vi "3.24版-复材超声C扫缺陷分析评定软件.vi"() -> ()   [LabVIEW 2018]
doc: "使用该模板构建用户界面事件处理设计模式。将模板应用于对话框及其它用户界面。用户也可创建并执行VI可按照与用户界面事件相同方式处理的用户定义事件。"
uses:
  <vilib>/Utility/NIReport.llb/Report Type.ctl
  <vilib>/addons/_office/_exclsub.llb/font.ctl
  <vilib>/Utility/NIReport.llb/HTML Report Image Alignment.ctl
  <vilib>/Utility/NIReport.llb/Append Report Text (str wrap).vi
  <vilib>/Utility/NIReport.llb/Append Image to Report (path wrap).vi
  <vilib>/addons/_office/word.llb/Word Easy Table (str).vi
  <vilib>/Utility/NIReport.llb/NI_report.lvclass
  <vilib>/vision/NI_Vision_Development_Module.lvlib
  <vilib>/Utility/NIReport.llb/Word/NI_Word.lvclass
  <vilib>/addons/_office/NI_ReportGenerationToolkit.lvlib
  <vilib>/Utility/NIReport.llb/NI_ReportGenerationCore.lvlib
panel:
  out "报告模式":string
  in  "删除标注":bool caption="定量分析"
  out "输入的灰度阈值":dbl caption="值"
  out "反射图原始路径":path
  out "穿透图原始路径":path
  out "ROImask":T1(plugin-control)
  out "模式选择":u16(ring) items=["只读穿透图", "穿透图和反射图结合"]
  out "添加的路径":path
  out "连接的字符串 2":string
  out "临界面积百分比值":dbl
  out "临界Z值":i32
  out "标注后的图片路径":path
  out "弥散类检测结果合并":string[][](table)
  out "分层类检测结果合并":string[][](table)
  out "弥散类检测结果":string[][](table)
  out "分层类检测结果":string[][](table)
  out "部位信息":string[](array[string])=["", "34.500000", "32.500000", "1121", "34", "54.955926", "分层类", "不合格", ""]
  out "连接的字符串":string
  out "框数":dbl
  out "自定义字体":T2={"Desired Font (Application)"=enum."Application Font", "[User-specified Font]"={"Font Name"="", "Size"=12, "Strikeout?"=FALSE, "Italic?"=FALSE, "Underline?"=FALSE, "Outline?"=FALSE, "Shadow?"=FALSE, "Bold?"=FALSE, "Rotation Angle"=0.0}, "Horizontal Alignment"=0, "Vertical Alignment"=0} {"Horizontal Alignment" items=["Left", "Center", "Right"]; "Vertical Alignment" items=["Bottom", "Top", "Baseline"]}
  out "框组":T3(array[cluster])
  out "质量等级":string
  out "灰度阈值":dbl
  in  "stop":bool caption="停止"
  in  "导入图像":bool caption="导入图片"
  in  "图像预处理":bool
  in  "自定义色彩":bool
  in  "开始标注":bool caption="定量分析"
  in  "查看标注":bool caption="辅助定性分析"
  in  "生成评定结果":bool caption="生成原始记录"
  in  "控件":enum32{"穿透图", "反射图"}(tab)
  out "穿透图":T1(plugin-control)
  out "反射图":T1(plugin-control)
  out "产品规格":cluster{"产品长度（周长）（mm）":dbl, "产品宽度（母线长）（mm）":dbl}
  out "图像分辨率":T4
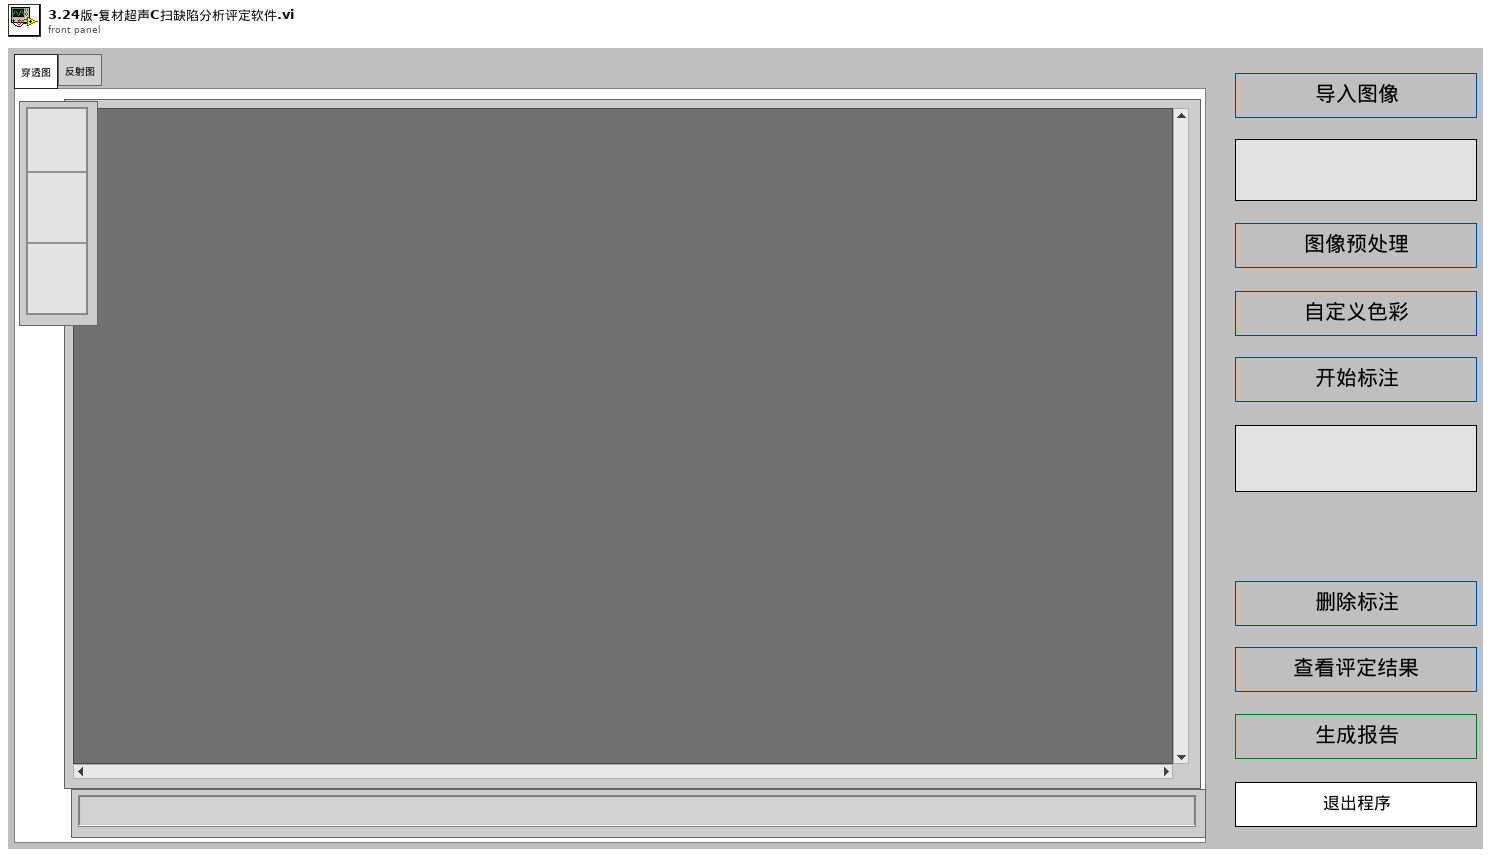
[diagram p1: front panel]
types:
  T1 = typedef "IMAQ Image.ctl" = refnum<image>
  T2 = cluster{"Desired Font (Application)":enum16{"User-specified Font", "Application Font", "System Font", "Dialog Font"}, "[User-specified Font]":cluster{"Font Name":string, "Size":i16, "Strikeout?":bool, "Italic?":bool, "Underline?":bool, "Outline?":bool, "Shadow?":bool, "Bold?":bool, "Rotation Angle":dbl}, "Horizontal Alignment":i16, "Vertical Alignment":i16}
  T3 = cluster{"Global Rectangle":i32[], "Contours":cluster{"Contour Type":u32, "ROI Type":u32, "Points":i32[]}[]}[]
  T4 = cluster{"图像X向分辨率（mm/像素）":dbl, "图像Y向分辨率（mm/像素）":dbl}
  T5 = cluster{"Global Rectangle":i32[], "Contours":cluster{"Contour Type":u32, "ROI Type":u32, "Points":i32[]}[]}
  T6 = cluster{"Zoom Tool":bool, "Selection Tool":bool, "Pan Tool":bool, "Point Tool":bool, "Line Tool":bool, "Rectangle Tool":bool, "Rotated Rectangle Tool":bool, "Polyline Tool":bool, "Polygon Tool":bool, "Freehand Tool":bool, "Closed Freehand Tool":bool, "Ellipse Tool":bool, "Annulus Tool":bool}
  T7 = enum8{"Enabled", "Disabled", "Disabled and Grayed Out"}
  T8 = enum32{"Invalid", "Standard", "Closed", "Hidden", "Minimized", "Maximized"}
  T9 = enum32{"Linear", "Log", "Exp", "Square", "Square root", "Power X", "Power 1/X"}
  T10 = enum32{"Gray", "Binary", "Gradient", "Rainbow", "Temperature"}
  T11 = enum16{"maximized", "minimized", "normal", "no change"}
  T12 = typedef "NI_ReportGenerationCore.lvlib/Report Type.ctl" = enum16{"HTML", "Word", "Excel"}
  T13 = typedef "NI_ReportGenerationCore.lvlib/HTML Report Image Alignment.ctl" = enum16{"(default)", "LEFT", "RIGHT", "TOP", "TEXTTOP", "MIDDLE", "ABSMIDDLE", "BASELINE", "BOTTOM", "ABSBOTTOM"}
  T14 = cluster{"position (Excel)":cluster{"row":i32, "column":i32}, "name (Excel)":string, "bookmark (Word)":string}
  T15 = cluster{"position (excel)":cluster{"row":i32, "column":i32}, "name (excel)":string, "bookmark (word)":string}
  T16 = typedef "NI_ReportGenerationToolkit.lvlib/font.ctl" = cluster{"font name":string, "font size":dbl, "bold":u16, "italic":u16, "underline":u16, "strike through":u16, "font color":u32}
  T17 = typedef "Image Type" = u32
  T18 = cluster{"Red (or Hue) value":u8, "Green (or Sat) value":u8, "Blue (or Light or Val) value":u8}[]
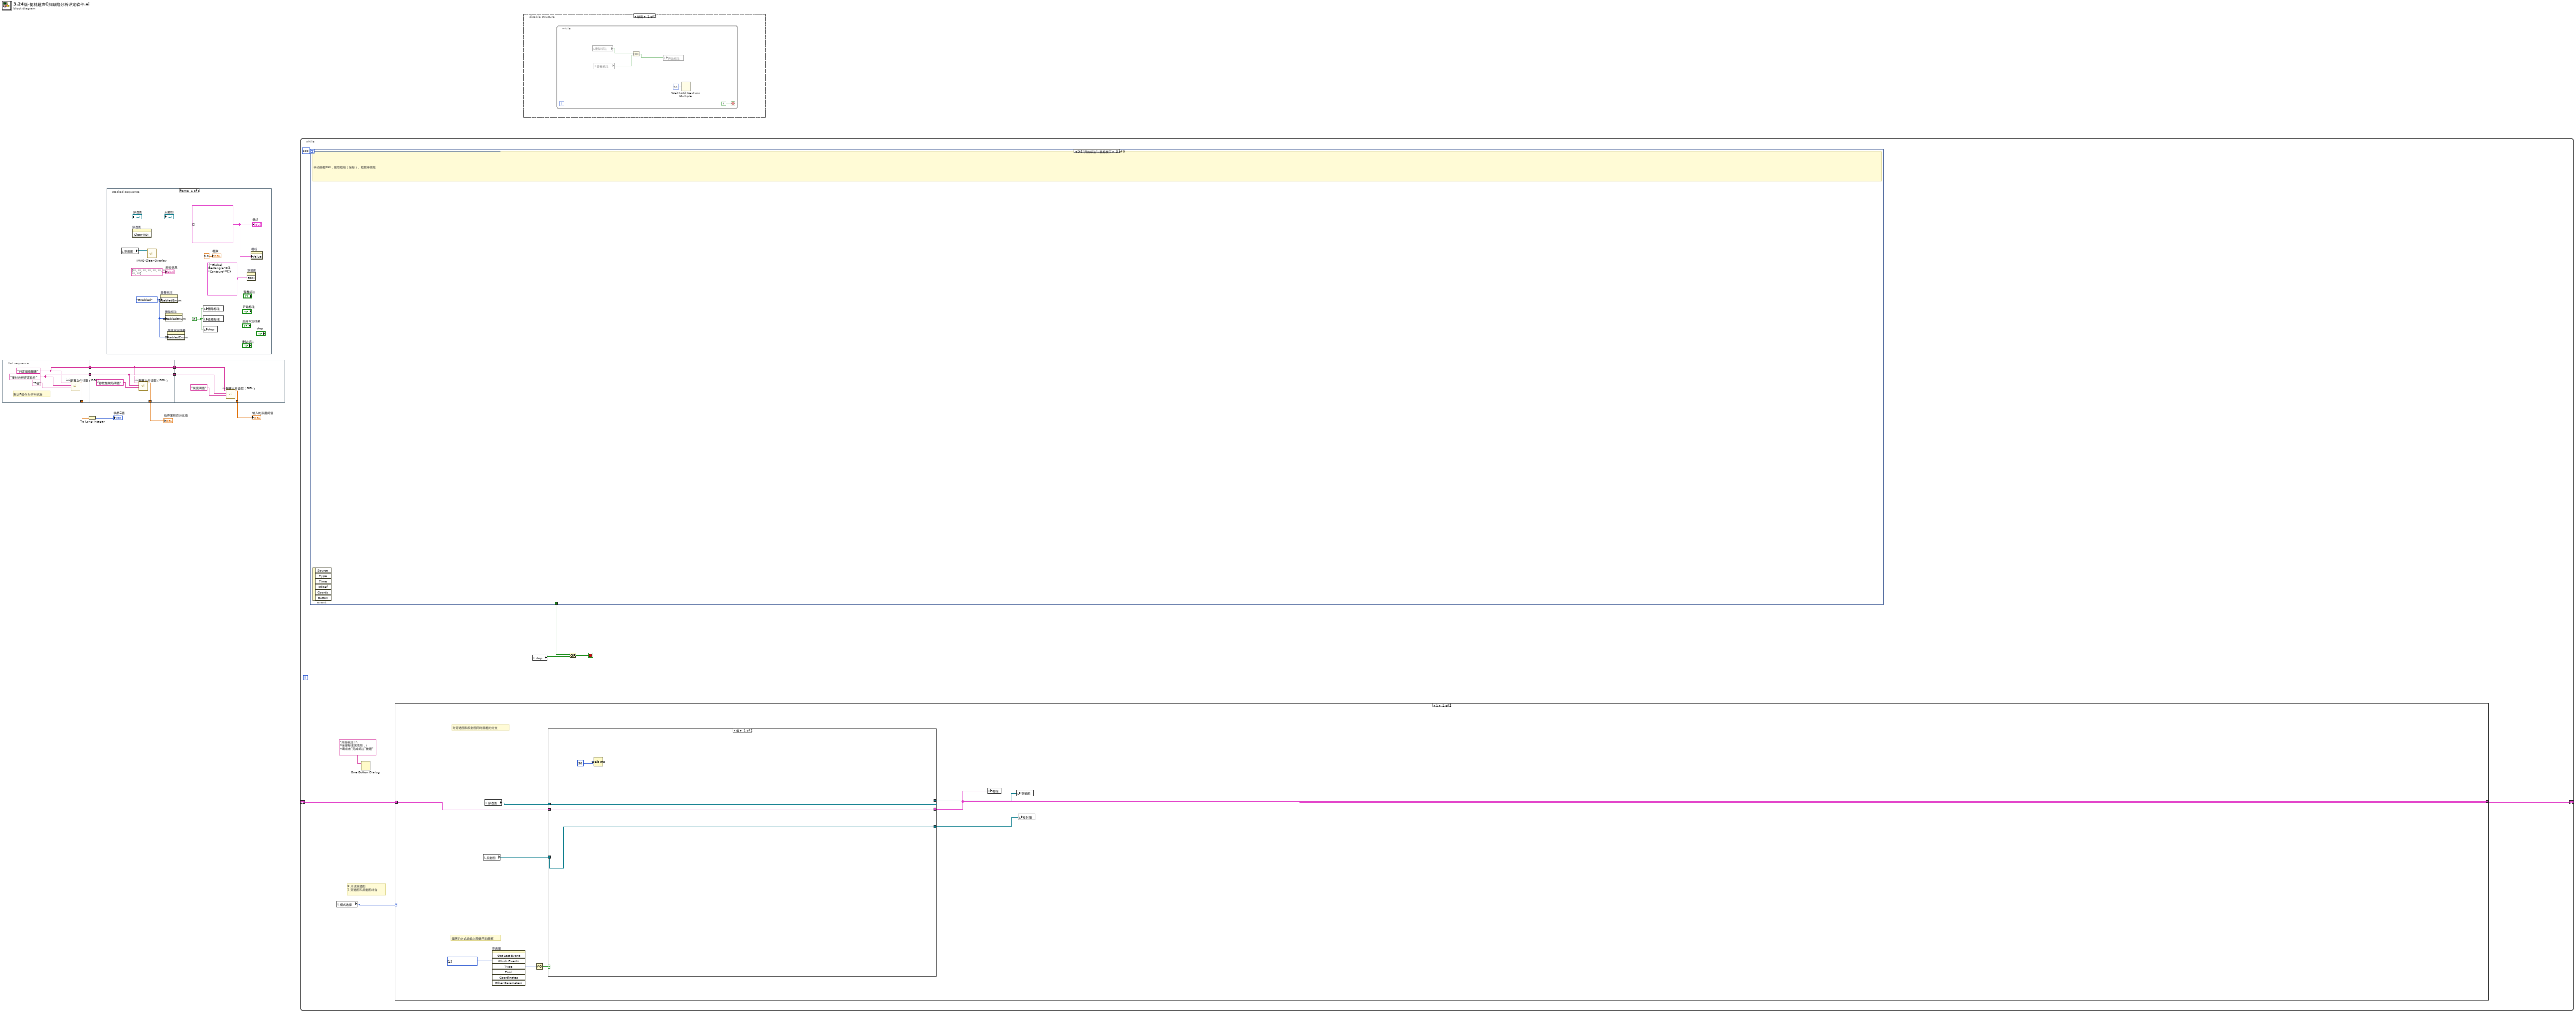
[diagram p0: block diagram]
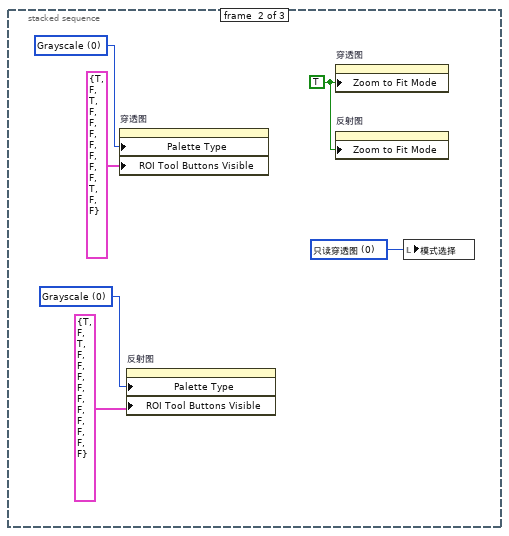
[diagram p2: hidden frame]
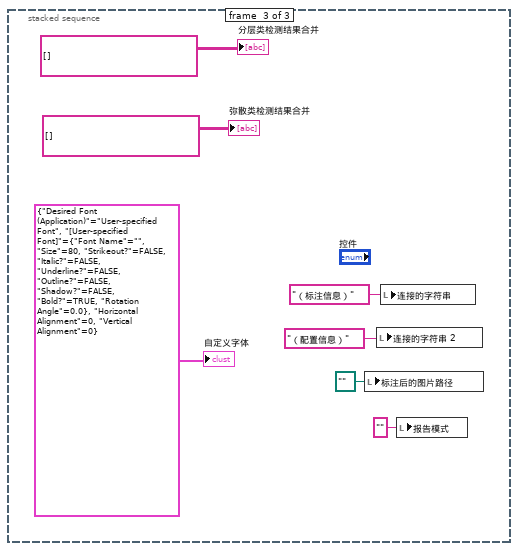
[diagram p3: hidden frame]
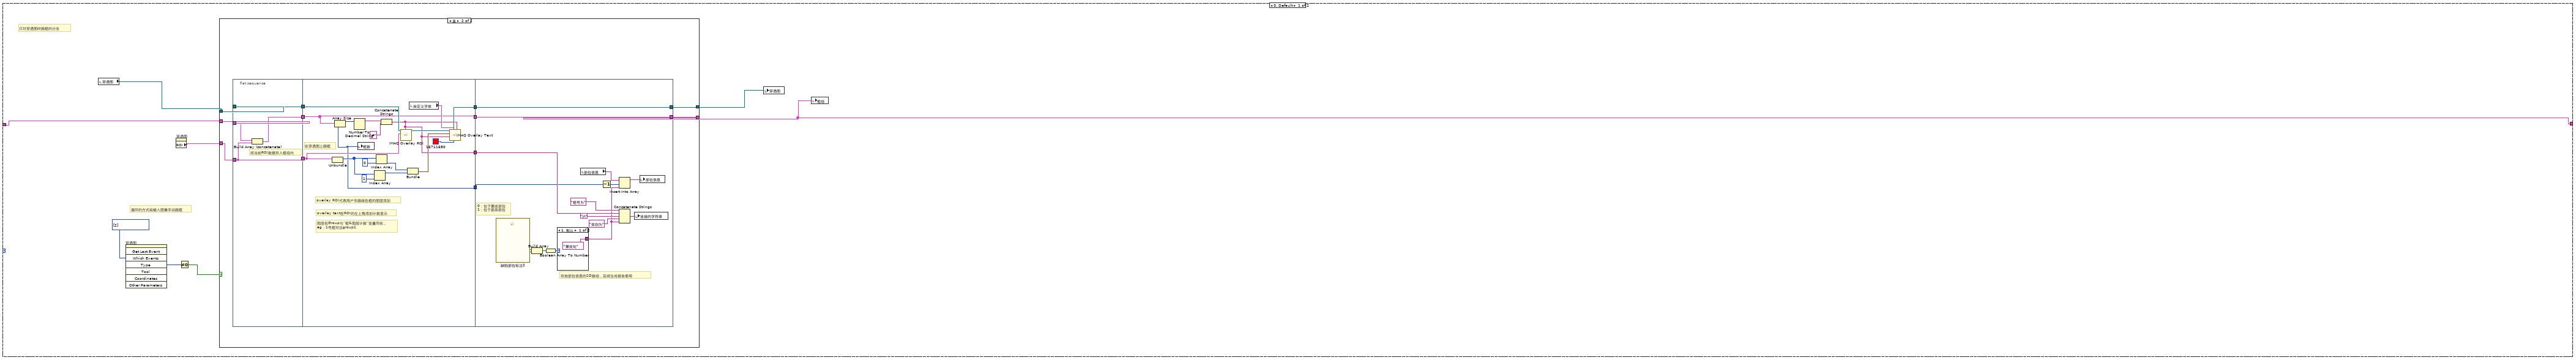
[diagram p5: hidden frame]
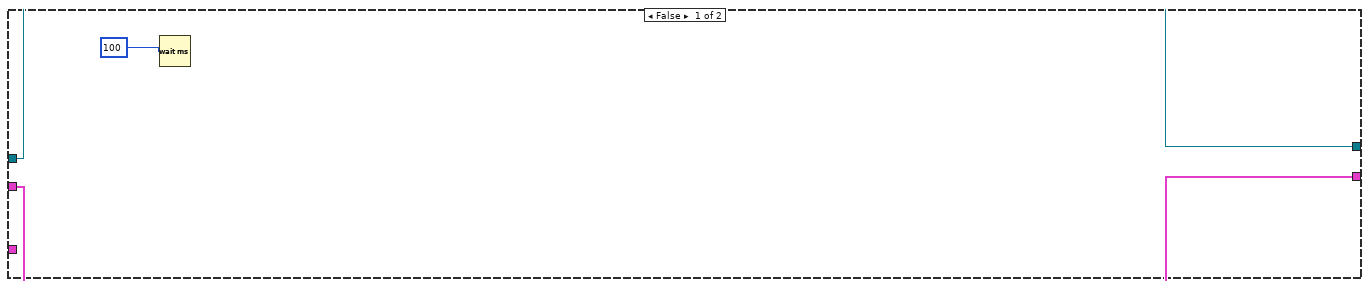
[diagram p6: hidden frame]
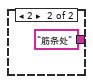
[diagram p7: hidden frame]
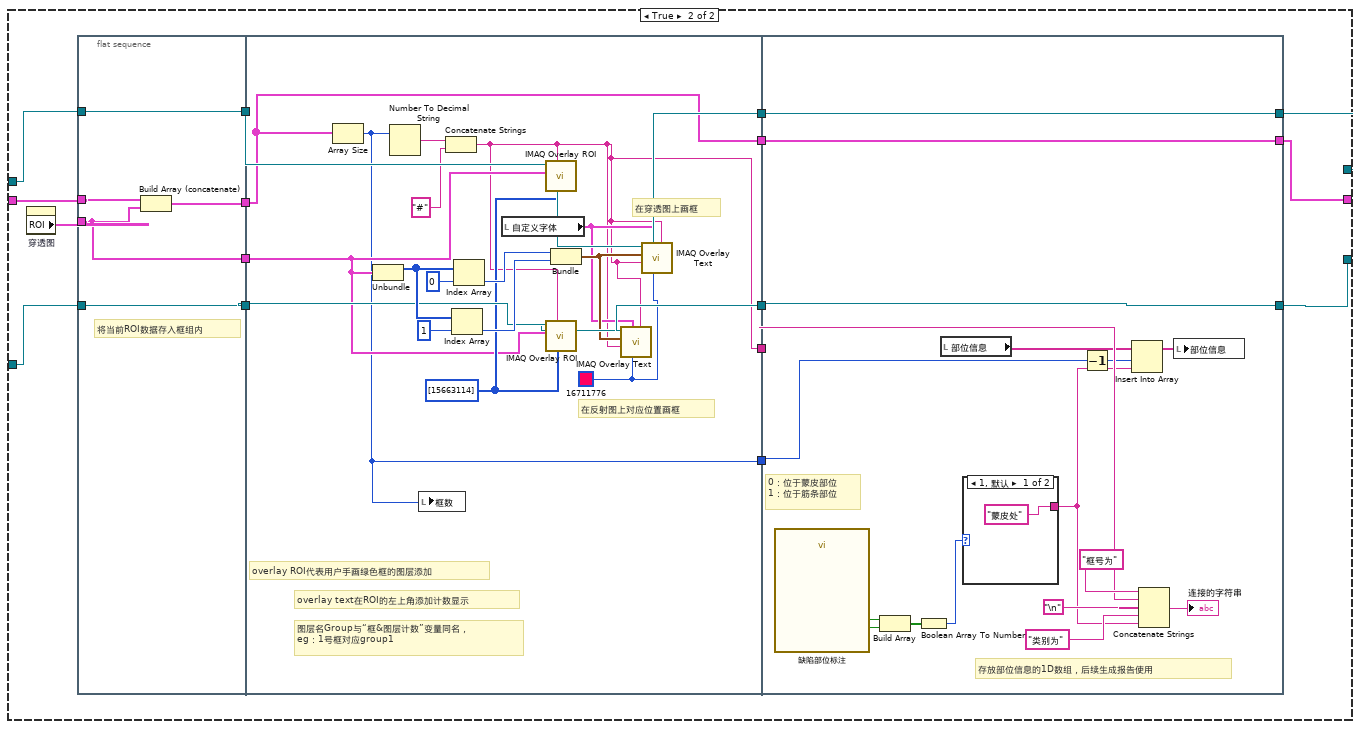
[diagram p8: hidden frame]
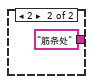
[diagram p9: hidden frame]
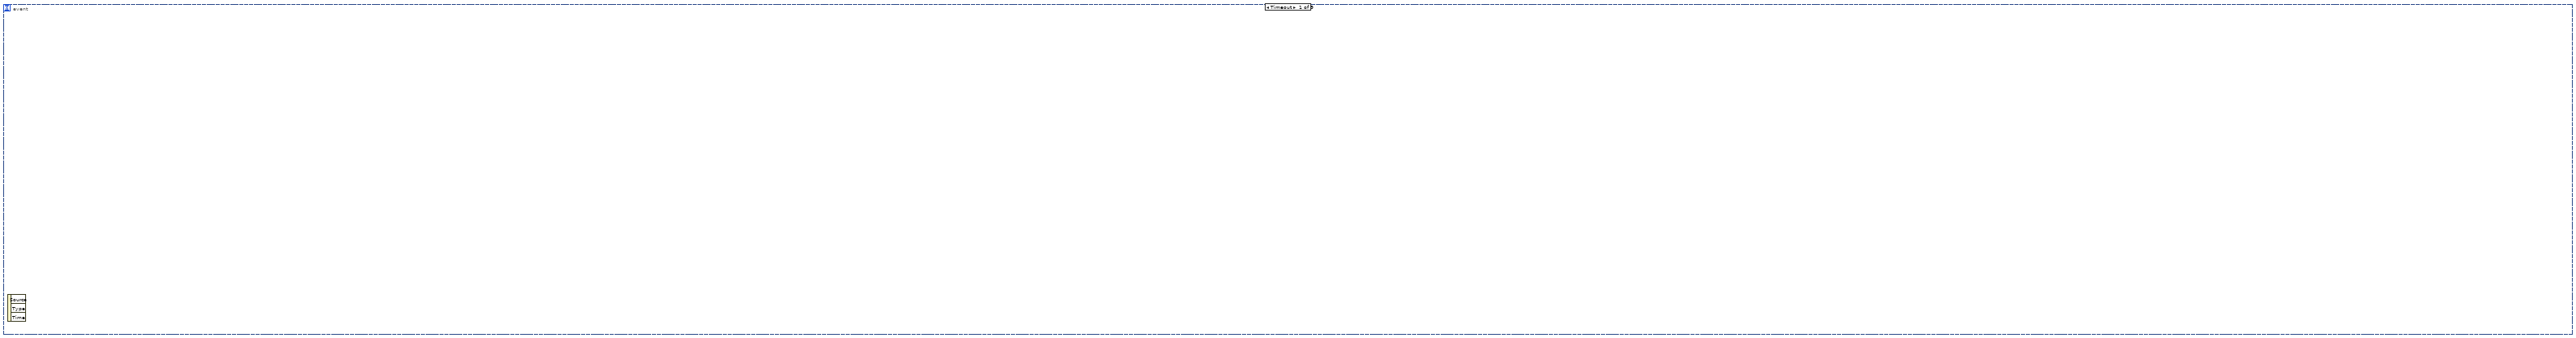
[diagram p10: hidden frame]
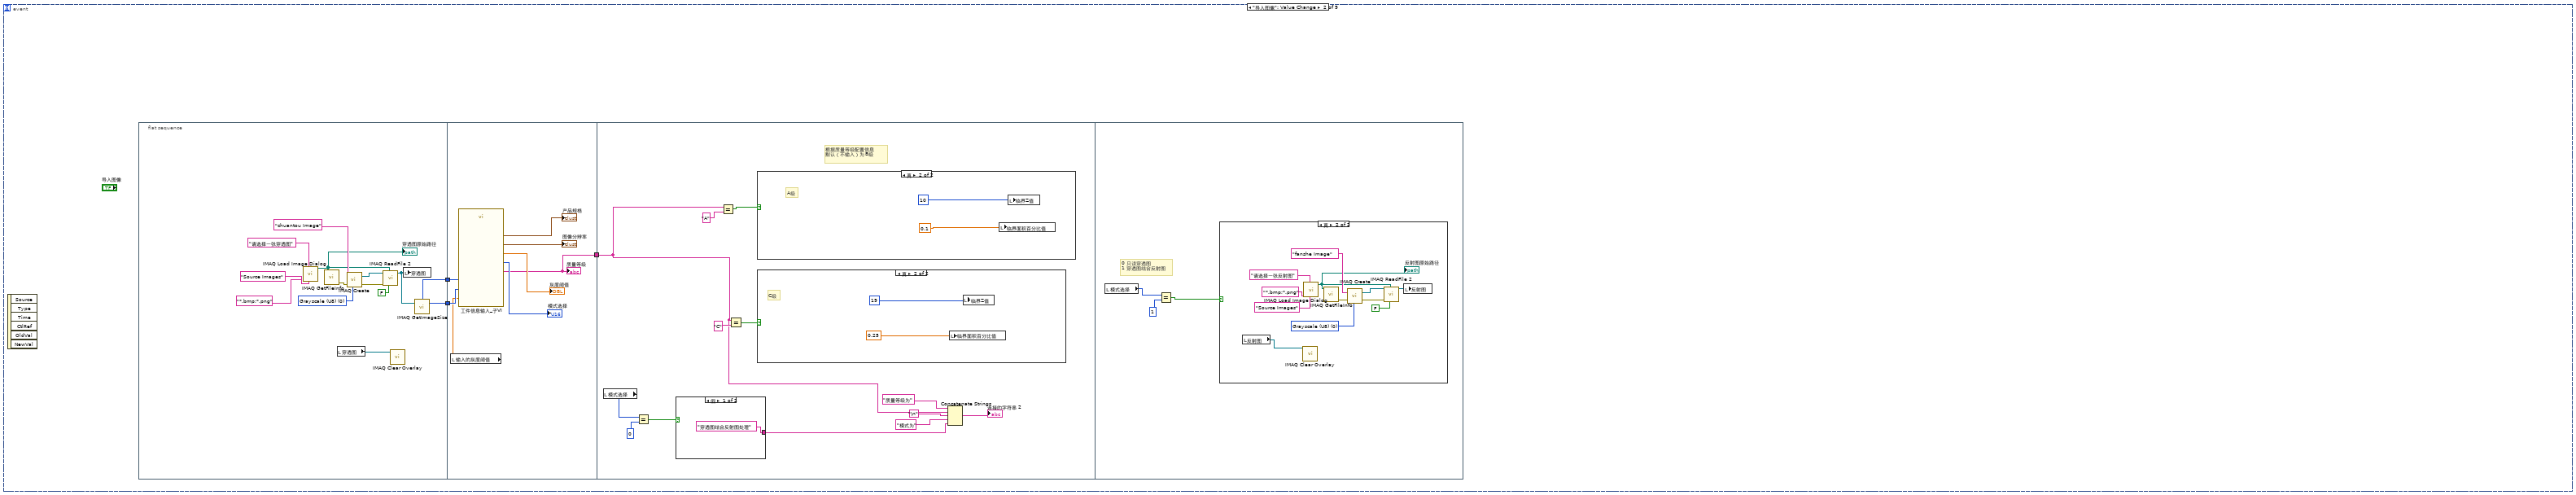
[diagram p11: hidden frame]
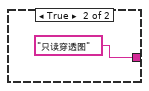
[diagram p12: hidden frame]
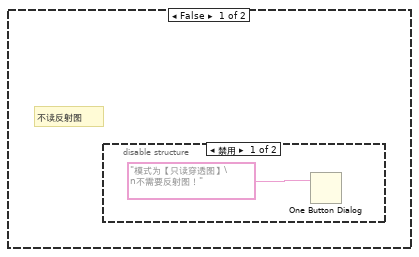
[diagram p15: hidden frame]
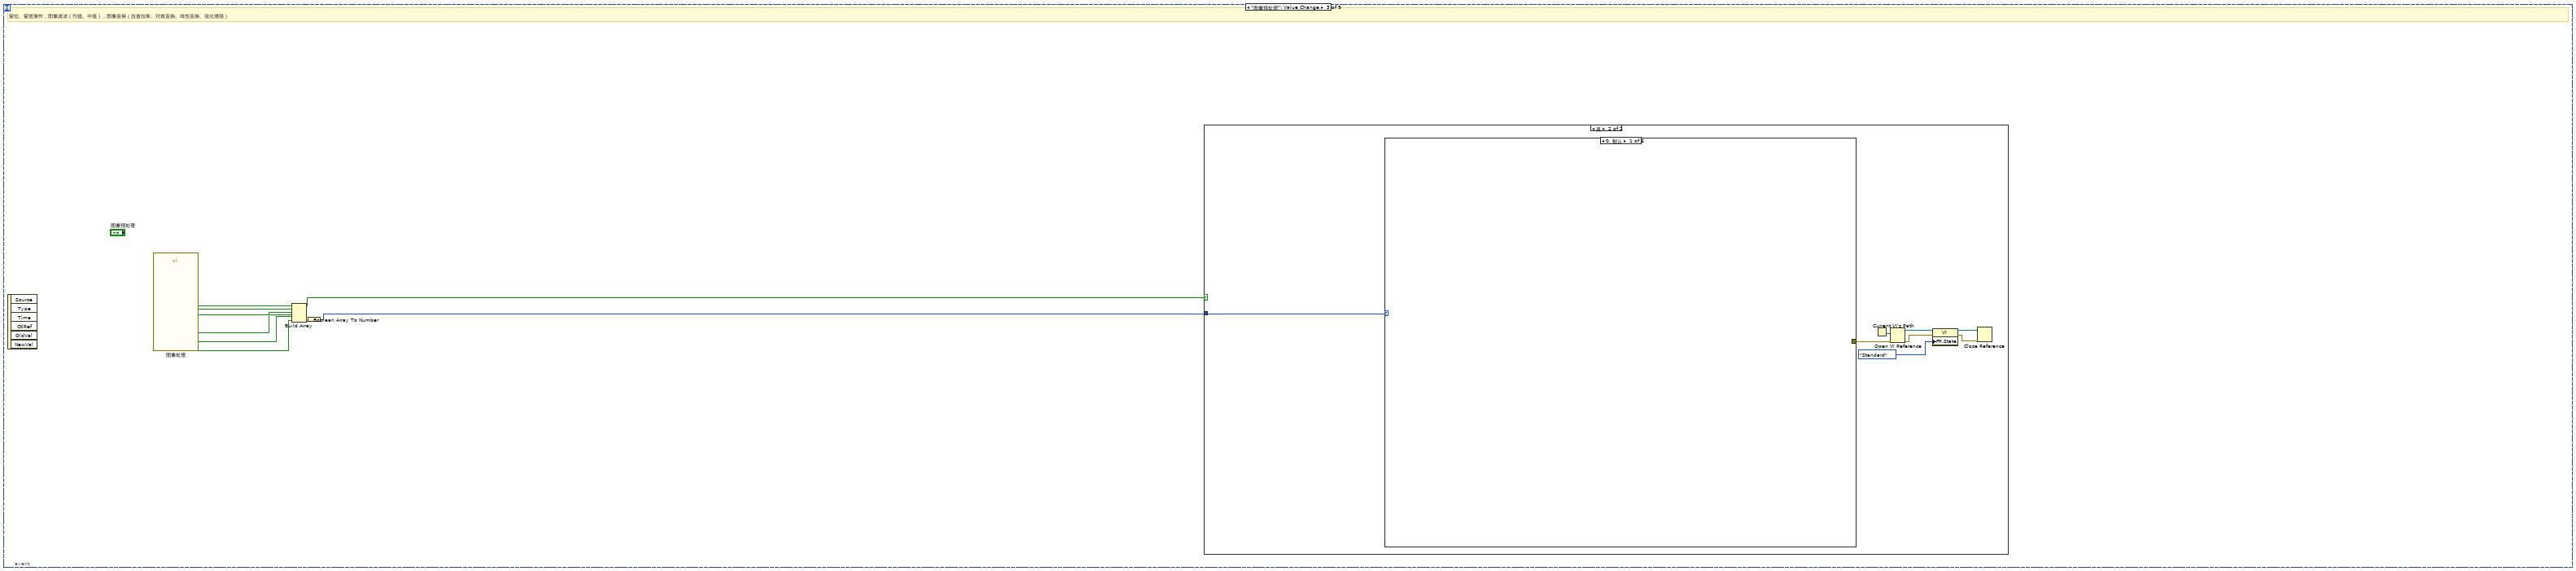
[diagram p17: hidden frame]
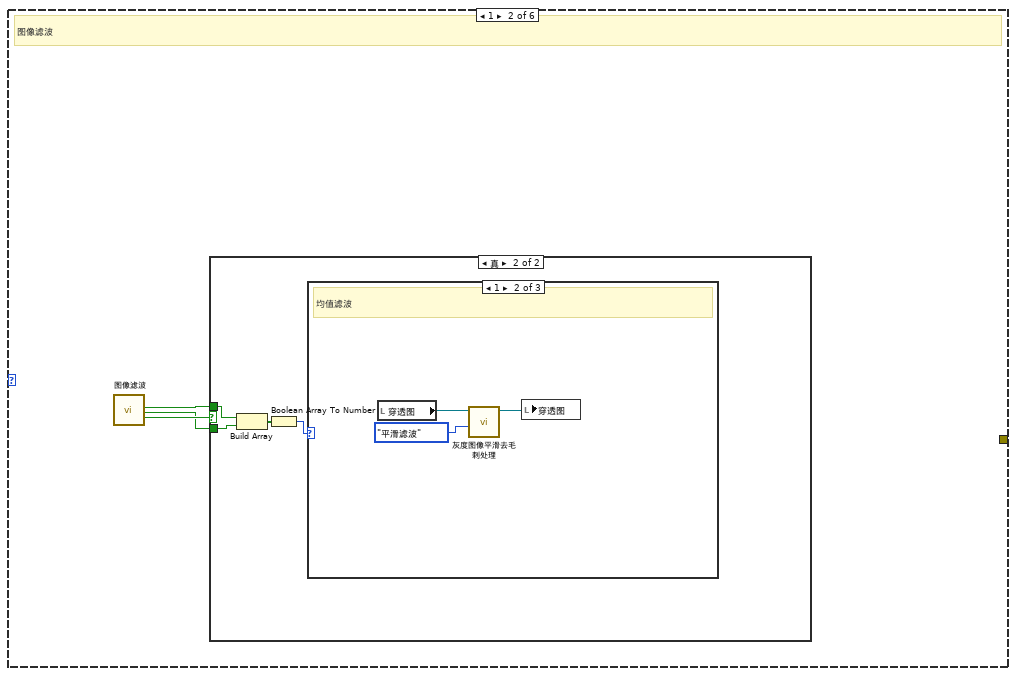
[diagram p19: hidden frame]
diagram:
  n1 = flat-sequence {
    tunnel: [w11] -> w8
    tunnel: [w10] -> w7
    tunnel: [w9] -> w2
    tunnel: w8 -> [w14]
    tunnel: w7 -> [w15]
    tunnel: [w15] -> w6
    tunnel: [w14] -> w5
    tunnel: [w13] -> w3
    tunnel: w6 -> [w19]
    tunnel: w5 -> [w18]
    tunnel: [w17] -> w4
    frame #0 {
      w10 = "复材分析评定软件" ("section")
      w11 = "判定阈值配置" ("文件名称")
      # "默认B级作为评判标准"
      n2 = call "ini配置文件读取（DBL）.vi"("key"="Z值", "section"=w10, "文件名称"=w11) -> ("value"=w9:dbl)  [unwired: 8 in]
    }
    frame #1 {
      n3 = call "ini配置文件读取（DBL）.vi"("key"="弥散性缺陷阈值", "section"=w15, "文件名称"=w14) -> ("value"=w13:dbl)  [unwired: 8 in]
    }
    frame #2 {
      n4 = call "ini配置文件读取（DBL）.vi"("key"="灰度阈值", "section"=w19, "文件名称"=w18) -> ("value"=w17:dbl)  [unwired: 8 in]
    }
  }
  n5 = To Long Integer(number=w2) -> (32bit integer=→"临界Z值":i32)
  n6 = stacked-sequence {
    frame #0 {
      w25 = T3 [] ("框组")
      w22 = T7."Enabled" ("禁用")
      w21 = FALSE ("查看标注")
      n7 = local read "穿透图"() -> (w23:T1)
      n8 = invoke on="穿透图" class="ImageControl" method="Clear ROI"() -> ()  [unwired: 3 in, 3 out]
      n9 = call "IMAQ Clear Overlay"("Image"=w23) -> ()  [unwired: 9 in, 2 out]
      n10 = property on="查看标注" class="Bool (严格)"("DisabledEnum"=w22) -> ()  [unwired: 2 in, 2 out]
      n11 = property on="删除标注" class="Bool (严格)"("DisabledEnum"=w22) -> ()  [unwired: 2 in, 2 out]
      n12 = property on="生成评定结果" class="Bool"("DisabledEnum"=w22) -> ()  [unwired: 2 in, 2 out]
      n13 = local write "删除标注"(w21) -> ()
      n14 = local write "查看标注"(w21) -> ()
      n15 = local write "stop"(w21) -> ()
      n16 = property on="穿透图" class="ImageControl"("ROI"=T5 {"Global Rectangle"=[], "Contours"=[]}) -> ()  [unwired: 2 in, 2 out]
      n17 = property on="框组" class="Arr (严格)"("Value"=w25) -> ()  [unwired: 2 in, 2 out]
      "部位信息" <- string[] ["", "", "", "", "", "", "", "", ""] ("部位信息")
      "框组" <- w25
      "框数" <- 0.0 ("框数")
    }
    frame #1 {
      w28 = u16 0 items=["只读穿透图", "穿透图和反射图结合"] ("模式选择")
      w30 = u32 0 items=["Grayscale", "Binary", "Gradient", "Rainbow", "Temperature", "User Defined", "Binary 16 Bit", "Gradient 16 Bit", "Rainbow 16 Bit", "Temperature 16 Bit", "User Defined 16 Bit"] ("Palette:Palette Type")
      w31 = TRUE ("Zoom to Fit Mode")
      w33 = u32 0 items=["Grayscale", "Binary", "Gradient", "Rainbow", "Temperature", "User Defined", "Binary 16 Bit", "Gradient 16 Bit", "Rainbow 16 Bit", "Temperature 16 Bit", "User Defined 16 Bit"] ("Palette:Palette Type")
      n18 = property on="穿透图" class="ImageControl"("Palette Type"=w33, "ROI Tool Buttons Visible"=T6 {"Zoom Tool"=TRUE, "Selection Tool"=FALSE, "Pan Tool"=TRUE, "Point Tool"=FALSE, "Line Tool"=FALSE, "Rectangle Tool"=FALSE, "Rotated Rectangle Tool"=FALSE, "Polyline Tool"=FALSE, "Polygon Tool"=FALSE, "Freehand Tool"=FALSE, "Closed Freehand Tool"=TRUE, "Ellipse Tool"=FALSE, "Annulus Tool"=FALSE} ("ROI Tool Buttons Visible:All Elements")) -> ()  [unwired: 2 in, 2 out]
      n19 = property on="反射图" class="ImageControl"("Palette Type"=w30, "ROI Tool Buttons Visible"=T6 {"Zoom Tool"=TRUE, "Selection Tool"=FALSE, "Pan Tool"=TRUE, "Point Tool"=FALSE, "Line Tool"=FALSE, "Rectangle Tool"=FALSE, "Rotated Rectangle Tool"=FALSE, "Polyline Tool"=FALSE, "Polygon Tool"=FALSE, "Freehand Tool"=FALSE, "Closed Freehand Tool"=FALSE, "Ellipse Tool"=FALSE, "Annulus Tool"=FALSE} ("ROI Tool Buttons Visible:All Elements")) -> ()  [unwired: 2 in, 2 out]
      n20 = property on="穿透图" class="ImageControl"("Zoom to Fit Mode"=w31) -> ()  [unwired: 2 in, 2 out]
      n21 = property on="反射图" class="ImageControl"("Zoom to Fit Mode"=w31) -> ()  [unwired: 2 in, 2 out]
      n22 = local write "模式选择"(w28) -> ()
    }
    frame #2 {
      n23 = local write "标注后的图片路径"(path "" ("标注后的图片路径")) -> ()
      n24 = local write "连接的字符串 2"("（配置信息）" ("连接的字符串 2")) -> ()
      n25 = local write "连接的字符串"("（标注信息）" ("连接的字符串")) -> ()
      n26 = local write "报告模式"("" ("报告模式")) -> ()
      "自定义字体" <- T2 {"Desired Font (Application)"=enum."User-specified Font", "[User-specified Font]"={"Font Name"="", "Size"=80, "Strikeout?"=FALSE, "Italic?"=FALSE, "Underline?"=FALSE, "Outline?"=FALSE, "Shadow?"=FALSE, "Bold?"=TRUE, "Rotation Angle"=0.0}, "Horizontal Alignment"=0, "Vertical Alignment"=0} ("Font, Size & Style")
      "分层类检测结果合并" <- string[][] [] ("弥散类检测结果合并")
      "弥散类检测结果合并" <- string[][] [] ("弥散类检测结果合并")
    }
  }
  n27 = while {
    shift-right: [w44] -> _
    shift-left: _ -> [w45]
    stop <- w41 stop-if-true
    # "0 只读穿透图\n1 穿透图和反射图结合"
    n28 = event shown="[4] \"开始标注\": 鼠标按下" {
      selector: _ -> [_ _ _ _ _ _ _ _ _]
      dyn-events: _ -> [_ _ _ _ _ _ _ _ _]
      timeout: 100 -> [_ _ _ _ _ _ _ _ _]
      tunnel: [_ _ _ _ _ _ _ _ w763] -> w42
      event Timeout {
        n29 = event-data() -> ()  [unwired: 1 in, 3 out]
      }
      event "导入图像": Value Change {
        n30 = event-data() -> ()  [unwired: 1 in, 6 out]
        n31 = flat-sequence {
          tunnel: [w191] -> w187
          tunnel: [w190] -> w186
          tunnel: [w206] -> w188
          tunnel: w187 -> [w205]
          tunnel: w186 -> [w204]
          tunnel: w188 -> [w215]
          frame #0 {
            w194 = T17 0 items=["Grayscale (U8)", "Grayscale (I16)", "Grayscale (SGL)", "Complex (CSG)", "RGB (U32)", "HSL (U32)", "RGB (U64)", "Grayscale (U16)"] ("Image Type")
            n32 = call "IMAQ Load Image Dialog"("Pattern Label"="Source Images", "Prompt"="请选择一张穿透图" ("prompt"), "Pattern"="*.bmp;*.png") -> ("Path"=w193:path)  [unwired: 6 in, 2 out]
            "穿透图原始路径" <- w193
            n33 = call "IMAQ GetFileInfo"("File Path"=w193) -> ("error out"=w197:errorcluster)  [unwired: 4 in, 6 out]
            n34 = local read "穿透图"() -> (w189:T1)
            n35 = call "IMAQ Create"("Image Name"="chuantou Image", "Image Type"=w194, "error in (no error)"=w197) -> ("New Image"=w198:T1, "error out"=w199:errorcluster)  [unwired: 2 in]
            n36 = call "IMAQ ReadFile 2"("Use File Path Image Type"=FALSE, "File Path"=w193, "error in (no error)"=w199, "Image"=w198) -> ("Image Out"=w192:T1)  [unwired: 3 in, 4 out]
            n37 = call "IMAQ Clear Overlay"("Image"=w189) -> ()  [unwired: 9 in, 2 out]
            n38 = local write "穿透图"(w192) -> ()
            n39 = call "IMAQ GetImageSize"("Image"=w192) -> ("Y Resolution"=w190:i32, "X Resolution"=w191:i32)  [unwired: 3 in, 1 out]
          }
          frame #1 {
            n40 = local read "输入的灰度阈值"() -> (w203:dbl)
            n41 = call "工件信息输入_子VI.vi"("Y Resolution"=w204, "X Resolution"=w205, "输入的灰度阈值"=w203) -> ("质量等级"=w206:string, "模式选择"=→"模式选择":u16, "灰度阈值"=→"灰度阈值":dbl, "产品规格"=→"产品规格":cluster{"产品长度（周长）（mm）":dbl, "产品宽度（母线长）（mm）":dbl}, "图像分辨率"=→"图像分辨率":T4)  [unwired: 3 in]
            "质量等级" <- w206
          }
          frame #2 {
            # "根据质量等级配置信息\n默认（不输入）为B级"
            n42 = local read "模式选择"() -> (w213:u16)
            n43 = Equal?(x=w213, y=u16 0) -> (x = y?=w212:bool)
            n44 = case shown="假" w212 {
              tunnel: ["穿透图结合反射图处理" ("字符串") "只读穿透图" ("字符串")] -> w211
              frame False {
              }
              frame True {
              }
            }
            n45 = Equal?(x=w215, y="A") -> (x = y?=w218:bool)
            n46 = Equal?(x=w215, y="C") -> (x = y?=w219:bool)
            n47 = case shown="真" w218 {
              frame False {
              }
              frame True {
                # "A级"
                n48 = local write "临界面积百分比值"(0.1 ("临界面积百分比值")) -> ()
                n49 = local write "临界Z值"(10 ("临界Z值")) -> ()
              }
            }
            n50 = case shown="真" w219 {
              frame False {
              }
              frame True {
                # "C级"
                n51 = local write "临界面积百分比值"(0.25 ("临界面积百分比值")) -> ()
                n52 = local write "临界Z值"(19 ("临界Z值")) -> ()
              }
            }
            n53 = Concatenate Strings("质量等级为" ("字符串"), w215, "\n", "模式为" ("字符串"), w211) -> (→"连接的字符串 2":string)
          }
          frame #3 {
            # "0 只读穿透图\n1 穿透图结合反射图"
            n54 = local read "模式选择"() -> (w231:u16)
            n55 = Equal?(x=w231, y=u16 1) -> (x = y?=w230:bool)
            n56 = case shown="真" w230 {
              frame False {
                # "不读反射图"
                n57 = disable-structure shown="禁用" {
                  frame Disabled {
                    n58 = One Button Dialog(message="模式为【只读穿透图】\n不需要反射图！" ("消息")) -> ()  [unwired: 1 in, 1 out]
                  }
                  frame Enabled {
                  }
                }
              }
              frame True {
                w237 = T17 0 items=["Grayscale (U8)", "Grayscale (I16)", "Grayscale (SGL)", "Complex (CSG)", "RGB (U32)", "HSL (U32)", "RGB (U64)", "Grayscale (U16)"] ("Image Type")
                n59 = local read "反射图"() -> (w234:T1)
                n60 = call "IMAQ Clear Overlay"("Image"=w234) -> ()  [unwired: 9 in, 2 out]
                n61 = call "IMAQ Load Image Dialog"("Pattern Label"="Source Images", "Prompt"="请选择一张反射图" ("prompt"), "Pattern"="*.bmp;*.png") -> ("Path"=w236:path)  [unwired: 6 in, 2 out]
                "反射图原始路径" <- w236
                n62 = call "IMAQ GetFileInfo"("File Path"=w236) -> ("error out"=w240:errorcluster)  [unwired: 4 in, 6 out]
                n63 = call "IMAQ Create"("Image Name"="fanshe Image", "Image Type"=w237, "error in (no error)"=w240) -> ("New Image"=w241:T1, "error out"=w242:errorcluster)  [unwired: 2 in]
                n64 = call "IMAQ ReadFile 2"("Use File Path Image Type"=FALSE, "File Path"=w236, "error in (no error)"=w242, "Image"=w241) -> ("Image Out"=w235:T1)  [unwired: 3 in, 4 out]
                n65 = local write "反射图"(w235) -> ()
              }
            }
          }
        }
      }
      event "图像预处理": Value Change {
        # "窗位、窗宽操作，图像滤波（均值、中值），图像变换（拉普拉斯、对数变换、线性变换、锐化增强）"
        n66 = event-data() -> ()  [unwired: 1 in, 6 out]
        n67 = call "图像处理"() -> ("撤销图像处理"=w246:bool, "线性灰度值测量"=w247:bool, "窗位窗宽"=w252:bool, "图像增强"=w248:bool, "图像滤波"=w253:bool, "确定"=w249:bool)  [unwired: 13 in, 1 out]
        n68 = Build Array(w253, w248, w252, w247, w246) -> (w251:bool[])
        n69 = Boolean Array To Number(Boolean array=w251) -> (number=w250:u32)
        n70 = case shown="真" w249 {
          tunnel: w250 -> [_ w261]
          frame False {
          }
          frame True {
            n71 = case shown="0, 默认" w261 {
              tunnel: [_ _ errorcluster {"status"=FALSE, "code"=0, "source"=""} ("错误输入（无错误）") _ _ _] -> w254
              frame 0, Default {
              }
              frame 1 {
                # "图像滤波"
                n72 = call "图像滤波"() -> ("均值滤波"=w263:bool, "中值滤波"=w262:bool, "确定"=w264:bool)  [unwired: 16 in, 1 out]
                n73 = case shown="真" w264 {
                  tunnel: w263 -> [_ w267]
                  tunnel: w262 -> [_ w266]
                  frame False {
                  }
                  frame True {
                    n74 = Build Array(w267, w266) -> (w268:bool[])
                    n75 = Boolean Array To Number(Boolean array=w268) -> (number=w265:u32)
                    n76 = case shown="1" w265 {
                      frame 0, Default {
                      }
                      frame 1 {
                        # "均值滤波"
                        n77 = local read "穿透图"() -> (w271:T1)
                        n78 = call "灰度图像平滑去毛刺处理.vi"("滤波方法选择"=enum16{"中值滤波", "平滑滤波"}."平滑滤波", "Image"=w271) -> ("Image Out"=w270:T1)  [unwired: 9 in]
                        n79 = local write "穿透图"(w270) -> ()
                      }
                      frame 2 {
                        # "中值滤波"
                        n80 = local read "穿透图"() -> (w274:T1)
                        n81 = call "灰度图像平滑去毛刺处理.vi"("滤波方法选择"=enum16{"中值滤波", "平滑滤波"}."中值滤波", "Image"=w274) -> ("Image Out"=w273:T1)  [unwired: 9 in]
                        n82 = local write "穿透图"(w273) -> ()
                      }
                    }
                  }
                }
              }
              frame 2 {
                # "图像增强"
                n83 = call "图像增强"() -> ("幂变换"=w276:bool, "阈值变换"=w277:bool, "高斯变换"=w278:bool, "指数变换"=w279:bool, "对数变换"=w280:bool, "确定"=w281:bool)  [unwired: 13 in, 1 out]
                n84 = case shown="真" w281 {
                  tunnel: w280 -> [_ w286]
                  tunnel: w279 -> [_ w285]
                  tunnel: w278 -> [_ w284]
                  tunnel: w277 -> [_ w283]
                  tunnel: w276 -> [_ w282]
                  frame False {
                  }
                  frame True {
                    n85 = Build Array(w286, w285, w284, w283, w282) -> (w288:bool[])
                    n86 = Boolean Array To Number(Boolean array=w288) -> (number=w287:u32)
                    n87 = case shown="2" w287 {
                      frame 0, Default {
                      }
                      frame 1 {
                        # "对数变换"
                        n88 = call "对数变换"() -> ("变换系数K"=w289:dbl, "确定"=w290:bool)  [unwired: 17 in, 1 out]
                        n89 = case shown="真" w290 {
                          tunnel: w289 -> [_ w291]
                          frame False {
                          }
                          frame True {
                            n90 = local read "穿透图"() -> (w295:T1)
                            n91 = call "IMAQ MathLookup"("Range"=cluster{"Minimum":sgl, "Maximum":sgl} {"Minimum"=0.0, "Maximum"=255.0}, "Operator"=T9."Log", "X Value"=w291, "Image Dst"=w295, "Image Src"=w295) -> ("Image Dst Out"=w293:T1)  [unwired: 5 in, 1 out]
                            n92 = local write "穿透图"(w293) -> ()
                          }
                        }
                      }
                      frame 2 {
                        # "指数变换"
                        n93 = call "指数变换"() -> ("变换系数K"=w296:dbl, "确定"=w297:bool)  [unwired: 17 in, 1 out]
                        n94 = case shown="真" w297 {
                          tunnel: w296 -> [_ w298]
                          frame False {
                          }
                          frame True {
                            n95 = local read "穿透图"() -> (w302:T1)
                            n96 = call "IMAQ MathLookup"("Range"=cluster{"Minimum":sgl, "Maximum":sgl} {"Minimum"=0.0, "Maximum"=255.0}, "Operator"=T9."Exp", "X Value"=w298, "Image Dst"=w302, "Image Src"=w302) -> ("Image Dst Out"=w300:T1)  [unwired: 5 in, 1 out]
                            n97 = local write "穿透图"(w300) -> ()
                          }
                        }
                      }
                      frame 4 {
                        w308 = u16 4 items=["Gradient"=1, "Laplacian"=2, "Smoothing"=3, "Gaussian"=4] ("Kernel Family")
                        # "高斯斯变换"
                        n98 = local read "穿透图"() -> (w305:T1)
                        n99 = call "IMAQ GetKernel"("Kernel Family"=w308, "Kernel Size (3,5,...)"=3) -> ("Kernel"=w306:sgl[][], "Divider"=w303:sgl)  [unwired: 6 in, 2 out]
                        n100 = call "IMAQ Convolute"("Kernel"=w306, "Divider (kernel sum)"=w303, "Image Dst"=w305, "Image Src"=w305) -> ("Image Dst Out"=w304:T1)  [unwired: 6 in, 1 out]
                        n101 = local write "穿透图"(w304) -> ()
                      }
                      frame 8 {
                        # "阈值变换"
                        n102 = call "阈值范围选择子VI.vi"() -> ("阈值范围"=w309:cluster{"Lower value":sgl, "Upper value":sgl}, "确定执行"=w310:bool)  [unwired: 10 in]
                        n103 = case shown="真" w310 {
                          tunnel: w309 -> [_ w312]
                          frame False {
                          }
                          frame True {
                            n104 = local read "穿透图"() -> (w315:T1)
                            n105 = call "IMAQ Threshold"("Replace Value"=sgl 255.0, "Keep/Replace Value (Replace)"=TRUE, "Range"=w312, "Image Dst"=w315, "Image Src"=w315) -> ("Image Dst Out"=w314:T1)  [unwired: 5 in, 1 out]
                            n106 = local write "穿透图"(w314) -> ()
                          }
                        }
                      }
                      frame 16 {
                        # "幂变换"
                        n107 = call "幂变换"() -> ("变换系数K"=w316:dbl, "确定"=w317:bool)  [unwired: 17 in, 1 out]
                        n108 = case shown="真" w317 {
                          tunnel: w316 -> [_ w318]
                          frame False {
                          }
                          frame True {
                            n109 = local read "穿透图"() -> (w322:T1)
                            n110 = call "IMAQ MathLookup"("Range"=cluster{"Minimum":sgl, "Maximum":sgl} {"Minimum"=0.0, "Maximum"=255.0}, "Operator"=T9."Power 1/X", "X Value"=w318, "Image Dst"=w322, "Image Src"=w322) -> ("Image Dst Out"=w320:T1)  [unwired: 5 in, 1 out]
                            n111 = local write "穿透图"(w320) -> ()
                          }
                        }
                      }
                    }
                  }
                }
              }
              frame 4 {
                # "窗位窗宽"
                n112 = Two Button Dialog(message="确定进行窗位窗宽操作？" ("消息")) -> (T button?=w324:bool)  [unwired: 2 in]
                n113 = case shown="真" w324 {
                  frame False {
                  }
                  frame True {
                    n114 = property on="穿透图" class="ImageControl"() -> (error out=w326:errorcluster, "Palette Type"=w333:u32)  [unwired: 2 in, 1 out]
                    n115 = Current VI's Path() -> (path=w328:path)
                    n116 = Open VI Reference(vi path=w328, error in (no error)=w326) -> (vi reference=w329:refnum<vi>, error out=w331:errorcluster)  [unwired: 4 in]
                    n117 = case shown="4" w333 {
                      tunnel: [w336 w338 w340 w342 w344] -> w334
                      frame 0, Default {
                        # "灰度"
                        n118 = call "IMAQ GetPalette"("Palette Number (gray)"=T10."Gray") -> ("Color Palette"=w336:cluster{"Red":u8, "Green":u8, "Blue":u8}[])  [unwired: 4 in, 1 out]
                      }
                      frame 2 {
                        # "梯度"
                        n119 = call "IMAQ GetPalette"("Palette Number (gray)"=T10."Gradient") -> ("Color Palette"=w338:cluster{"Red":u8, "Green":u8, "Blue":u8}[])  [unwired: 4 in, 1 out]
                      }
                      frame 3 {
                        # "彩虹"
                        n120 = call "IMAQ GetPalette"("Palette Number (gray)"=T10."Rainbow") -> ("Color Palette"=w340:cluster{"Red":u8, "Green":u8, "Blue":u8}[])  [unwired: 4 in, 1 out]
                      }
                      frame 4 {
                        # "温度"
                        n121 = call "IMAQ GetPalette"("Palette Number (gray)"=T10."Temperature") -> ("Color Palette"=w342:cluster{"Red":u8, "Green":u8, "Blue":u8}[])  [unwired: 4 in, 1 out]
                      }
                      frame 5 {
                        # "自定义"
                        n122 = property on="穿透图" class="ImageControl"() -> ("User Palette"=w344:cluster{"Red":u8, "Green":u8, "Blue":u8}[])  [unwired: 2 in, 2 out]
                      }
                    }
                    n123 = property class="VI"(reference=w329, error in=w331, "FP.State"=T8."Hidden" ("前面板窗口:状态")) -> (reference out=w330:refnum<vi>, error out=w332:errorcluster)
                    n124 = Close Reference(reference=w330, error in (no error)=w332) -> ()  [unwired: 1 out]
                    n125 = local read "穿透图"() -> (w325:T1)
                    n126 = call "窗位窗宽调整子VI.vi"("Image in"=w325, "Palette:User Palette"=w334, "Palette:Palette Type"=w333) -> ("Image out"=w335:T1)  [unwired: 8 in]
                    n127 = local write "穿透图"(w335) -> ()
                  }
                }
              }
              frame 8 {
                # "查看线灰度值曲线，用于精确测量"
                n128 = Current VI's Path() -> (path=w351:path)
                n129 = Open VI Reference(vi path=w351) -> (vi reference=w350:refnum<vi>, error out=w348:errorcluster)  [unwired: 5 in]
                n130 = property class="VI"(reference=w350, error in=w348, "FP.State"=T8."Hidden" ("前面板窗口:状态")) -> (reference out=w349:refnum<vi>, error out=w347:errorcluster)
                n131 = Close Reference(reference=w349, error in (no error)=w347) -> (error out=w345:errorcluster)
                n132 = case shown="无错误" w345 {
                  frame No Error {
                    n133 = property on="穿透图" class="ImageControl"() -> ("Palette Type"=w353:u32)  [unwired: 2 in, 2 out]
                    n134 = case shown="2" w353 {
                      tunnel: [w356 w358 w360 w362 w364] -> w352
                      frame 0, Default {
                        # "灰度"
                        n135 = call "IMAQ GetPalette"("Palette Number (gray)"=T10."Gray") -> ("Color Palette"=w356:cluster{"Red":u8, "Green":u8, "Blue":u8}[])  [unwired: 4 in, 1 out]
                      }
                      frame 2 {
                        # "梯度"
                        n136 = call "IMAQ GetPalette"("Palette Number (gray)"=T10."Gradient") -> ("Color Palette"=w358:cluster{"Red":u8, "Green":u8, "Blue":u8}[])  [unwired: 4 in, 1 out]
                      }
                      frame 3 {
                        # "彩虹"
                        n137 = call "IMAQ GetPalette"("Palette Number (gray)"=T10."Rainbow") -> ("Color Palette"=w360:cluster{"Red":u8, "Green":u8, "Blue":u8}[])  [unwired: 4 in, 1 out]
                      }
                      frame 4 {
                        # "温度"
                        n138 = call "IMAQ GetPalette"("Palette Number (gray)"=T10."Temperature") -> ("Color Palette"=w362:cluster{"Red":u8, "Green":u8, "Blue":u8}[])  [unwired: 4 in, 1 out]
                      }
                      frame 5 {
                        # "自定义"
                        n139 = property on="穿透图" class="ImageControl"() -> ("User Palette"=w364:cluster{"Red":u8, "Green":u8, "Blue":u8}[])  [unwired: 2 in, 2 out]
                      }
                    }
                    n140 = local read "穿透图"() -> (w355:T1)
                    n141 = local read "图像分辨率"() -> (w354:T4)
                    n142 = call "线性灰度值曲线查看子VI.vi"("Palette:User Palette"=w352, "图像分辨率"=w354, "Image"=w355) -> ()  [unwired: 9 in]
                  }
                  frame Error {
                  }
                }
              }
              frame 16 {
                # "撤销图像处理，恢复原图"
                n143 = call "IMAQ Create"("Image Name"="P1") -> ("New Image"=w365:T1)  [unwired: 4 in, 1 out]
                n144 = local write "穿透图"(w365) -> ()
              }
            }
            n145 = Current VI's Path() -> (path=w260:path)
            n146 = Open VI Reference(vi path=w260, error in (no error)=w254) -> (vi reference=w259:refnum<vi>, error out=w256:errorcluster)  [unwired: 4 in]
            n147 = property class="VI"(reference=w259, error in=w256, "FP.State"=T8."Standard" ("前面板窗口:状态")) -> (reference out=w257:refnum<vi>, error out=w255:errorcluster)
            n148 = Close Reference(reference=w257, error in (no error)=w255) -> ()  [unwired: 1 out]
          }
        }
      }
      event "自定义色彩": Value Change {
        # "色彩、色阶自定义"
        n149 = event-data() -> ()  [unwired: 1 in, 6 out]
        n150 = call "调色板"() -> ("自定义显示"=w368:bool, "温度显示"=w369:bool, "彩虹显示"=w370:bool, "梯度显示"=w371:bool, "灰度显示"=w372:bool, "确定"=w373:bool)  [unwired: 13 in, 1 out]
        n151 = Build Array(w372, w371, w370, w369, w368) -> (w367:bool[])
        n152 = case shown="真" w373 {
          tunnel: w367 -> [_ w376]
          frame False {
          }
          frame True {
            n153 = Boolean Array To Number(Boolean array=w376) -> (number=w375:u32)
            n154 = case shown="0, 默认" w375 {
              tunnel: [w377 w378 w379 w380 w381 w383] -> w374
              frame 0, Default {
                w377 = u32 0 items=["Grayscale", "Binary", "Gradient", "Rainbow", "Temperature", "User Defined", "Binary 16 Bit", "Gradient 16 Bit", "Rainbow 16 Bit", "Temperature 16 Bit", "User Defined 16 Bit"] ("Palette:Palette Type")
              }
              frame 1 {
                w378 = u32 0 items=["Grayscale", "Binary", "Gradient", "Rainbow", "Temperature", "User Defined", "Binary 16 Bit", "Gradient 16 Bit", "Rainbow 16 Bit", "Temperature 16 Bit", "User Defined 16 Bit"] ("Palette:Palette Type")
                # "灰度"
              }
              frame 2 {
                w379 = u32 2 items=["Grayscale", "Binary", "Gradient", "Rainbow", "Temperature", "User Defined", "Binary 16 Bit", "Gradient 16 Bit", "Rainbow 16 Bit", "Temperature 16 Bit", "User Defined 16 Bit"] ("Palette:Palette Type")
                # "梯度"
              }
              frame 4 {
                w380 = u32 3 items=["Grayscale", "Binary", "Gradient", "Rainbow", "Temperature", "User Defined", "Binary 16 Bit", "Gradient 16 Bit", "Rainbow 16 Bit", "Temperature 16 Bit", "User Defined 16 Bit"] ("Palette:Palette Type")
                # "彩虹"
              }
              frame 8 {
                w381 = u32 4 items=["Grayscale", "Binary", "Gradient", "Rainbow", "Temperature", "User Defined", "Binary 16 Bit", "Gradient 16 Bit", "Rainbow 16 Bit", "Temperature 16 Bit", "User Defined 16 Bit"] ("Palette:Palette Type")
                # "温度"
              }
              frame 16 {
                w383 = u32 5 items=["Grayscale", "Binary", "Gradient", "Rainbow", "Temperature", "User Defined", "Binary 16 Bit", "Gradient 16 Bit", "Rainbow 16 Bit", "Temperature 16 Bit", "User Defined 16 Bit"] ("Palette:Palette Type")
                # "自定义"
                n155 = call "自定义成像色谱20200214.vi"() -> ("Color palette"=w382:T18)  [unwired: 8 in, 1 out]
                n156 = property on="穿透图" class="ImageControl"("User Palette"=w382) -> ()  [unwired: 2 in, 2 out]
              }
            }
            n157 = property on="穿透图" class="ImageControl"("Palette Type"=w374) -> ()  [unwired: 2 in, 2 out]
          }
        }
      }
      event "开始标注": Mouse Down {
        # "手动画框ROI，提取框组（坐标）、框数等信息"
        n158 = event-data() -> ()  [unwired: 1 in, 6 out]
      }
      event "删除标注": Value Change {
        n159 = event-data() -> ()  [unwired: 1 in, 6 out]
        n160 = call "用户输入2"() -> ("框号"=w384:dbl, "确定"=w385:bool)  [unwired: 17 in, 1 out]
        n161 = case shown="真" w385 {
          tunnel: w384 -> [_ w386]
          frame False {
            # "用户取消操作"
          }
          frame True {
            n162 = stacked-sequence {
              tunnel: w386 -> [_ w393 _]
              frame #0 {
                # "1. 删除所有框"
                n163 = local read "穿透图"() -> (w387:T1)
                n164 = call "IMAQ Clear Overlay"("Image"=w387) -> ()  [unwired: 9 in, 2 out]
              }
              frame #1 {
                # "2. 删除框组中指定元素"
                n165 = local read "部位信息"() -> (w390:string[])
                n166 = local read "框组"() -> (w392:T3)
                n167 = Decrement(x=w393) -> (x-1=w389:dbl)
                n168 = Delete From Array(array=w390, index=w389) -> (array with subset deleted=w388:string[])  [unwired: 1 in, 1 out]
                n169 = Delete From Array(array=w392, index=w389) -> (array with subset deleted=w391:T3)  [unwired: 1 in, 1 out]
                n170 = local write "框组"(w391) -> ()
                n171 = local write "部位信息"(w388) -> ()
              }
              frame #2 {
                # "3. 重画所有框"
                n172 = while {
                  i -> [w406]
                  stop <- w397 stop-if-true
                  n173 = local read "框组"() -> (w401:T3)
                  n174 = local read "穿透图"() -> (w405:T1)
                  n175 = Array Size(array=w401) -> (size(s)=w402:i32)
                  n176 = Index Array(array=w401, index=w406) -> (element=w396:T5)
                  n177 = Increment(x=w406) -> (x+1=w413:i32)
                  n178 = local write "框数"(w402) -> ()
                  n179 = Greater Or Equal?(x=w413, y=w402) -> (x >= y?=w397:bool)
                  n180 = call "IMAQ Overlay ROI"("ROI Descriptor"=w396, "Image"=w405) -> ("Image Out"=w411:T1)  [unwired: 8 in, 1 out]
                  n181 = Unbundle(w396) -> ("Global Rectangle"=w403:i32[])  [unwired: 1 out]
                  n182 = Number To Decimal String(number=w413) -> (decimal integer string=w398:string)  [unwired: 1 in]
                  n183 = Index Array(array=w403, index=0 ("索引")) -> (element=w408:i32)
                  n184 = Index Array(array=w403, index=1 ("索引")) -> (element=w409:i32)
                  n185 = local read "自定义字体"() -> (w395:T2)
                  n186 = Concatenate Strings(w398, "#" ("字符串")) -> (w394:string)
                  n187 = Bundle(w408, w409) -> (w399:cluster{i32, i32})  [unwired: 1 in]
                  n188 = call "IMAQ Overlay Text"("Text Color (black)"=u32 16711680, "Font, Size & Style"=w395, "String"=w394, "Origin"=w399, "Image"=w411) -> ("Image Out"=w404:T1)  [unwired: 5 in, 1 out]
                  n189 = local write "穿透图"(w404) -> ()
                }
              }
            }
          }
        }
      }
      event "查看标注": Value Change {
        # "查看指定框的详细信息，包括灰度和面积阈值分割后的结果，提取到的长宽面积等信息"
        n190 = event-data() -> ()  [unwired: 1 in, 6 out]
        n191 = local read "模式选择"() -> (w423:u16)
        n192 = local read "临界面积百分比值"() -> (w417:dbl)
        n193 = local read "穿透图原始路径"() -> (w420:path)
        n194 = local read "临界Z值"() -> (w418:i32)
        n195 = local read "灰度阈值"() -> (w414:dbl)
        n196 = local read "部位信息"() -> (w422:string[])
        n197 = local read "产品规格"() -> (w421:cluster{"产品长度（周长）（mm）":dbl, "产品宽度（母线长）（mm）":dbl})
        n198 = local read "框组"() -> (w419:T3)
        n199 = case shown="1" w423 {
          tunnel: w422 -> [w433 w443]
          tunnel: w421 -> [w432 w442]
          tunnel: w420 -> [w431 w441]
          tunnel: w419 -> [w430 w440]
          tunnel: w418 -> [w429 w439]
          tunnel: w417 -> [w428 w438]
          tunnel: [w425 w437] -> w416
          tunnel: [w426 w436] -> w415
          tunnel: w414 -> [w427 w435]
          frame 0, Default {
            # "只读穿透图的图像处理方法"
            n200 = call "子界面-查看某框-只读穿透图模式.vi"("输入框号"=0.0 ("框号"), "框组"=w430, "临界Z值"=w429, "临界面积百分比值"=w428, "预先配置的灰度阈值"=w427, "穿透图原始路径"=w431, "部位信息"=w433, "产品规格"=w432) -> ("弥散类检测结果"=w425:string[][], "分层类检测结果"=w426:string[][])  [unwired: 10 in]
          }
          frame 1 {
            # "穿透图和反射图结合的图像处理方法"
            n201 = local read "反射图原始路径"() -> (w444:path)
            n202 = call "子界面-查看某框.vi"("输入框号"=0.0 ("框号"), "框组"=w440, "临界Z值"=w439, "反射图原始路径"=w444, "临界面积百分比值"=w438, "预先配置的灰度阈值"=w435, "穿透图原始路径"=w441, "部位信息"=w443, "产品规格"=w442) -> ("弥散类检测结果"=w437:string[][], "分层类检测结果"=w436:string[][])  [unwired: 9 in]
          }
        }
        "弥散类检测结果" <- w416
        "分层类检测结果" <- w415
      }
      event "生成评定结果": Value Change {
        # "相当于“查看标注”一栏中的操作做循环，遍历所有框，\n将输出结果叠加为数组，作为最终结果输出并导入word"
        n203 = event-data() -> ()  [unwired: 1 in, 6 out]
        n204 = call "报告模式选择"() -> ("自动检测结果"=w445:bool, "手动框选结果"=w446:bool)  [unwired: 16 in, 2 out]
        n205 = local read "分层类检测结果合并"() -> (w462:string[][])
        n206 = local read "弥散类检测结果合并"() -> (w460:string[][])
        n207 = Build Array(w446, w445) -> (w448:bool[])
        n208 = local read "模式选择"() -> (w469:u16)
        n209 = local read "临界面积百分比值"() -> (w463:dbl)
        n210 = local read "穿透图原始路径"() -> (w466:path)
        n211 = local read "灰度阈值"() -> (w461:dbl)
        n212 = Boolean Array To Number(Boolean array=w448) -> (number=w447:u32)
        n213 = local read "临界Z值"() -> (w464:i32)
        n214 = local read "产品规格"() -> (w467:cluster{"产品长度（周长）（mm）":dbl, "产品宽度（母线长）（mm）":dbl})
        n215 = local read "部位信息"() -> (w468:string[])
        n216 = local read "框组"() -> (w465:T3)
        n217 = case shown="2" w447 {
          tunnel: [w476 w545 w617] -> w473
          tunnel: [w475 w544 w616] -> w472
          tunnel: w469 -> [w481 w552 w622]
          tunnel: w468 -> [w479 w555 w625]
          tunnel: w467 -> [w478 w554 w624]
          tunnel: w466 -> [w480 w553 w623]
          tunnel: w465 -> [w482 w551 w621]
          tunnel: w464 -> [w484 w548 w620]
          tunnel: w463 -> [w485 w549 w619]
          tunnel: w462 -> [w487 w547 w615]
          tunnel: w461 -> [w483 w550 w618]
          tunnel: w460 -> [w486 w546 w614]
          frame 0, Default {
            # "默认手动框选结果"
            n218 = local read "框数"() -> (w477:dbl)
            n219 = case shown="0, 默认" w481 {
              tunnel: [w499 w527] -> w476
              tunnel: [w498 w526] -> w475
              tunnel: w487 -> [w489 w525]
              tunnel: w486 -> [w488 w524]
              tunnel: w485 -> [w492 w523]
              tunnel: w484 -> [w490 w522]
              tunnel: w483 -> [w491 w521]
              tunnel: w482 -> [w493 w520]
              tunnel: w480 -> [w494 w519]
              tunnel: w479 -> [w496 w518]
              tunnel: w478 -> [w495 w517]
              tunnel: w477 -> [w497 w516]
              frame 0, Default {
                # "只读穿透图的图像处理方法"
                n220 = for {
                  N: w497 -> [_]
                  shift-right: [w513] -> w499
                  shift-left: w489 -> [w512]
                  shift-right: [w507] -> w498
                  shift-left: w488 -> [w508]
                  tunnel: w496 -> [w506]
                  tunnel: w495 -> [w505]
                  tunnel: w494 -> [w504]
                  tunnel: w493 -> [w503]
                  tunnel: w492 -> [w502]
                  tunnel: w491 -> [w501]
                  tunnel: w490 -> [w500]
                  i -> [w511]
                  n221 = Increment(x=w511) -> (x+1=w510:i32)
                  n222 = call "子界面-查看某框-不显示界面-只读穿透图模式.vi"("框号"=w510, "框组"=w503, "临界Z值"=w500, "临界面积百分比值"=w502, "预先配置的灰度阈值"=w501, "穿透图原始路径"=w504, "部位信息"=w506, "产品规格"=w505) -> ("弥散类检测结果"=w509:string[][], "分层类检测结果"=w514:string[][])  [unwired: 10 in]
                  n223 = Build Array (concatenate)(w508, w509) -> (w507:string[][])
                  n224 = Build Array (concatenate)(w512, w514) -> (w513:string[][])
                }
              }
              frame 1 {
                # "穿透图和反射图结合的图像处理方法"
                n225 = local read "反射图原始路径"() -> (w515:path)
                n226 = for {
                  N: w516 -> [_]
                  shift-right: [w539] -> w527
                  shift-left: w525 -> [w541]
                  shift-right: [w538] -> w526
                  shift-left: w524 -> [w536]
                  tunnel: w523 -> [w535]
                  tunnel: w522 -> [w534]
                  tunnel: w521 -> [w533]
                  tunnel: w520 -> [w532]
                  tunnel: w519 -> [w529]
                  tunnel: w518 -> [w531]
                  tunnel: w517 -> [w530]
                  tunnel: w515 -> [w528]
                  i -> [w543]
                  n227 = Increment(x=w543) -> (x+1=w542:i32)
                  n228 = call "子界面-查看某框-不显示界面.vi"("框号"=w542, "框组"=w532, "临界Z值"=w534, "反射图原始路径"=w528, "临界面积百分比值"=w535, "预先配置的灰度阈值"=w533, "穿透图原始路径"=w529, "部位信息"=w531, "产品规格"=w530) -> ("弥散类检测结果"=w537:string[][], "分层类检测结果"=w540:string[][])  [unwired: 9 in]
                  n229 = Build Array (concatenate)(w541, w540) -> (w539:string[][])
                  n230 = Build Array (concatenate)(w536, w537) -> (w538:string[][])
                }
              }
            }
            "报告模式" <- "手动框选"
          }
          frame 1 {
            n231 = local read "框数"() -> (w556:dbl)
            n232 = local write "报告模式"("手动框选") -> ()
            n233 = case shown="1" w552 {
              tunnel: [w569 w597] -> w545
              tunnel: [w568 w596] -> w544
              tunnel: w556 -> [w567 w595]
              tunnel: w555 -> [w566 w594]
              tunnel: w554 -> [w565 w593]
              tunnel: w553 -> [w564 w592]
              tunnel: w551 -> [w563 w590]
              tunnel: w550 -> [w562 w589]
              tunnel: w549 -> [w561 w588]
              tunnel: w548 -> [w560 w591]
              tunnel: w547 -> [w559 w586]
              tunnel: w546 -> [w558 w585]
              frame 0, Default {
                # "只读穿透图的图像处理方法"
                n234 = for {
                  N: w567 -> [_]
                  shift-right: [w583] -> w569
                  shift-left: w559 -> [w582]
                  shift-right: [w577] -> w568
                  shift-left: w558 -> [w578]
                  tunnel: w566 -> [w576]
                  tunnel: w565 -> [w575]
                  tunnel: w564 -> [w574]
                  tunnel: w563 -> [w573]
                  tunnel: w562 -> [w572]
                  tunnel: w561 -> [w571]
                  tunnel: w560 -> [w570]
                  i -> [w581]
                  n235 = Increment(x=w581) -> (x+1=w580:i32)
                  n236 = call "子界面-查看某框-不显示界面-只读穿透图模式.vi"("框号"=w580, "框组"=w573, "临界Z值"=w570, "临界面积百分比值"=w571, "预先配置的灰度阈值"=w572, "穿透图原始路径"=w574, "部位信息"=w576, "产品规格"=w575) -> ("弥散类检测结果"=w579:string[][], "分层类检测结果"=w584:string[][])  [unwired: 10 in]
                  n237 = Build Array (concatenate)(w578, w579) -> (w577:string[][])
                  n238 = Build Array (concatenate)(w582, w584) -> (w583:string[][])
                }
              }
              frame 1 {
                # "穿透图和反射图结合的图像处理方法"
                n239 = local read "反射图原始路径"() -> (w587:path)
                n240 = for {
                  N: w595 -> [_]
                  shift-right: [w609] -> w597
                  shift-left: w586 -> [w611]
                  shift-right: [w608] -> w596
                  shift-left: w585 -> [w606]
                  tunnel: w594 -> [w605]
                  tunnel: w593 -> [w604]
                  tunnel: w592 -> [w603]
                  tunnel: w591 -> [w602]
                  tunnel: w590 -> [w601]
                  tunnel: w589 -> [w600]
                  tunnel: w588 -> [w599]
                  tunnel: w587 -> [w598]
                  i -> [w613]
                  n241 = Increment(x=w613) -> (x+1=w612:i32)
                  n242 = call "子界面-查看某框-不显示界面.vi"("框号"=w612, "框组"=w601, "临界Z值"=w602, "反射图原始路径"=w598, "临界面积百分比值"=w599, "预先配置的灰度阈值"=w600, "穿透图原始路径"=w603, "部位信息"=w605, "产品规格"=w604) -> ("弥散类检测结果"=w607:string[][], "分层类检测结果"=w610:string[][])  [unwired: 9 in]
                  n243 = Build Array (concatenate)(w611, w610) -> (w609:string[][])
                  n244 = Build Array (concatenate)(w606, w607) -> (w608:string[][])
                }
              }
            }
          }
          frame 2 {
            n245 = local write "报告模式"("自动检测") -> ()
            n246 = case shown="0, 默认" w622 {
              tunnel: [w640 w655] -> w617
              tunnel: [w639 w654] -> w616
              tunnel: w625 -> [w635 w650]
              tunnel: w624 -> [w634 w649]
              tunnel: w623 -> [w633 w648]
              tunnel: w621 -> [w632 w646]
              tunnel: w620 -> [w631 w643]
              tunnel: w619 -> [w630 w644]
              tunnel: w618 -> [w629 w645]
              tunnel: w615 -> [w628 w642]
              tunnel: w614 -> [w627 w641]
              frame 0, Default {
                # "只读穿透图的图像处理方法"
                n247 = call "子界面-查看某框-不显示界面-只读穿透图模式.vi"("框号"=0.0, "框组"=w632, "临界Z值"=w631, "临界面积百分比值"=w630, "预先配置的灰度阈值"=w629, "穿透图原始路径"=w633, "部位信息"=w635, "产品规格"=w634) -> ("弥散类检测结果"=w637:string[][], "分层类检测结果"=w638:string[][])  [unwired: 10 in]
                n248 = Build Array (concatenate)(w627, w637) -> (w639:string[][])
                n249 = Build Array (concatenate)(w628, w638) -> (w640:string[][])
              }
              frame 1 {
                # "穿透图和反射图结合的图像处理方法"
                n250 = local read "反射图原始路径"() -> (w647:path)
                n251 = call "子界面-查看某框-不显示界面.vi"("框号"=0.0, "框组"=w646, "临界Z值"=w643, "反射图原始路径"=w647, "临界面积百分比值"=w644, "预先配置的灰度阈值"=w645, "穿透图原始路径"=w648, "部位信息"=w650, "产品规格"=w649) -> ("弥散类检测结果"=w652:string[][], "分层类检测结果"=w653:string[][])  [unwired: 9 in]
                n252 = Build Array (concatenate)(w642, w653) -> (w655:string[][])
                n253 = Build Array (concatenate)(w641, w652) -> (w654:string[][])
              }
            }
          }
        }
        n254 = local write "弥散类检测结果合并"(w472) -> ()
        n255 = local write "分层类检测结果合并"(w473) -> ()
        n256 = flat-sequence {
          tunnel: w472 -> [w656]
          tunnel: w473 -> [w657]
          tunnel: [w657] -> w452
          tunnel: [w656] -> w450
          tunnel: w452 -> [w697]
          tunnel: [w697] -> w451
          tunnel: w450 -> [w696]
          tunnel: [w696] -> w449
          tunnel: w451 -> [w704]
          tunnel: w449 -> [w703]
          tunnel: [w704] -> w459
          tunnel: [w703] -> w458
          tunnel: [w702] -> w456
          tunnel: [w701] -> w455
          tunnel: [w724] -> w471
          tunnel: [w723] -> w470
          tunnel: w459 -> [w714]
          tunnel: w458 -> [w717]
          tunnel: [w717] -> w457
          tunnel: w456 -> [w716]
          tunnel: w455 -> [w715]
          tunnel: w471 -> [w736]
          tunnel: w470 -> [w735]
          tunnel: w457 -> [w734]
          tunnel: [w733] -> w454
          tunnel: [w732] -> w453
          tunnel: w454 -> [w755]
          tunnel: w453 -> [w754]
          frame #0 {
            n257 = while {
              tunnel: [w674] -> _
              i -> [w676]
              stop <- w674 stop-if-true
              w681 = 1 items=["White", "Black", "Inverted", "Black on White", "White on Black"] ("Color")
              w683 = u16 2 items=["Frame", "Paint", "Invert Frame", "Invert Paint"] ("Draw Mode")
              w678 = u16 1 items=["Line", "Rectangle", "Oval"] ("Shape to draw")
              # "生成绘制了ROI的图像\n可以用于后续的图片导出保存"
              n258 = local read "框组"() -> (w675:T3)
              n259 = local read "ROImask"() -> (w671:T1)
              n260 = local read "穿透图"() -> (w672:T1)
              n261 = Array Size(array=w675) -> (size(s)=w684:i32)
              n262 = Index Array(array=w675, index=w676) -> (element=w669:T5)
              n263 = Unbundle By Name(w669) -> ("Global Rectangle"=w664:i32[])
              n264 = Increment(x=w676) -> (x+1=w685:i32)
              n265 = Greater Or Equal?(x=w685, y=w684) -> (x >= y?=w674:bool)
              n266 = Index Array(array=w664, index=2 ("索引")) -> (element=w663:i32)
              n267 = Index Array(array=w664, index=0 ("索引")) -> (element=w660:i32)
              n268 = Index Array(array=w664, index=3 ("索引")) -> (element=w662:i32)
              n269 = Index Array(array=w664, index=1 ("索引")) -> (element=w659:i32)
              n270 = Number To Decimal String(number=w685) -> (decimal integer string=w679:string)  [unwired: 1 in]
              n271 = Build Array(w660, w659, w663, w662) -> (w661:i32[])
              n272 = call "IMAQ Draw"("Draw Mode"=w683, "Shape to draw"=w678, "Coordinates"=w661, "Image Src"=w672) -> ("Image Dst Out"=w682:T1)  [unwired: 6 in, 1 out]
              n273 = Concatenate Strings(w679, "#" ("字符串")) -> (w677:string)
              n274 = local read "自定义字体"() -> (w673:T2)
              n275 = Build Array(w660, w659) -> (w658:i32[])
              n276 = call "IMAQ Draw Text"("String"=w677, "Insertion Point"=w658, "Color"=w681, "Font, Size & Style"=w673, "Image Dst"=w671, "Image Src"=w682) -> ("Image Dst Out"=w670:T1)  [unwired: 2 in, 3 out]
              "ROImask" <- w670
              n277 = local write "ROImask"(w670) -> ()
            }
          }
          frame #1 {
            n278 = local read "穿透图原始路径"() -> (w695:path)
            n279 = local read "ROImask"() -> (w686:T1)
            n280 = Path To String(path=w695) -> (string=w692:string)
            n281 = String Length(string=w692) -> (length=w693:i32)
            n282 = Subtract(x=w693, y=4) -> (x-y=w694:i32)
            n283 = Replace Substring(3:w694, 4:"_标注后.png" ("字符串"), 5:w692) -> (1:w691:string)  [unwired: 1 in, 1 out]
            n284 = String To Path(string=w691) -> (path=w687:path)
            "标注后的图片路径" <- w687
            n285 = call-poly "IMAQ Write File 2"("Image Quality"=u32 1000, "File Path"=w687, "Image"=w686) -> ()  [unwired: 7 in, 2 out]
          }
          frame #2 {
            # "最终检测结果全部合并 导入word中"
            n286 = call <vilib>:"Application Directory.vi"() -> ("Application Directory"=w700:path)
            n287 = Build Path(base path=w700, name or relative path="report-template.docx") -> (appended path=w698:path)
            n288 = call <vilib>:"Create Report.vi"("window state (normal)"=T11."maximized", "report type"=Report_Type."Word", "template (empty)"=w698) -> ("report out"=w702:refnum<class "NI_report.lvclass">, "error out"=w701:errorcluster)  [unwired: 11 in]
          }
          frame #3 {
            n289 = Get Date/Time String(date format (0)=enum16{"short", "long", "abbreviated"}."long" ("日期格式(0)")) -> (date string=w721:string, time string=w722:string)  [unwired: 2 in]
            n290 = local read "标注后的图片路径"() -> (w712:path)
            n291 = Concatenate Strings(w721, w722) -> (w720:string)
            n292 = call-poly <vilib>:"Append Report Text.vi"("report in"=w716, "MS Office parameters"=T15 {"position (excel)"={"row"=0, "column"=0}, "name (excel)"="", "bookmark (word)"="time"}, "text"=w720, "error in (no error)"=w715) -> ("report out"=w711:refnum<class "NI_report.lvclass">, "error out"=w709:errorcluster)  [unwired: 8 in, 2 out]
            n293 = call-poly <vilib>:"Append Image to Report.vi"("report in"=w711, "alignment (default)"=HTML_Report_Image_Alignment."MIDDLE", "MS Office parameters"=T14 {"position (Excel)"={"row"=0, "column"=0}, "name (Excel)"="", "bookmark (Word)"="image"}, "path or URL of image"=w712, "error in (no error)"=w709) -> ("report out"=w708:refnum<class "NI_report.lvclass">, "error out"=w707:errorcluster)  [unwired: 7 in, 2 out]
            n294 = case shown="错误" w707 {
              frame No Error {
              }
              frame Error {
                n295 = One Button Dialog(message="图片导入word\n发生错误！" ("消息")) -> ()  [unwired: 1 in, 1 out]
              }
            }
            n296 = call <vilib>:"Word Easy Text.vi"("report in"=w708, "text"="分层类", "alignment (left)"=enum16{"Left", "Centered", "Right", "Justify"}."Left", "font"=T16 {"font name"="", "font size"=0.0, "bold"=0, "italic"=0, "underline"=0, "strike through"=0, "font color"=16777216}, "error in (no error)"=w707) -> ("report out"=w726:refnum<class "NI_report.lvclass">, "error out"=w727:errorcluster)  [unwired: 8 in, 1 out]
            n297 = call-poly <vilib>:"Word Easy Table.vi"("report in"=w726, "column headers"=string[] ["框号", "长/mm", "宽/mm", "面积/mm2", "Z值/mm", "部位", "类型", "合格性"], "data"=w714, "error in (no error)"=w727) -> ("report out"=w724:refnum<class "NI_report.lvclass">, "error out"=w723:errorcluster)  [unwired: 9 in, 1 out]
          }
          frame #4 {
            n298 = call <vilib>:"Word Easy Text.vi"("report in"=w736, "text"="弥散类", "alignment (left)"=enum16{"Left", "Centered", "Right", "Justify"}."Left", "font"=T16 {"font name"="", "font size"=0.0, "bold"=0, "italic"=0, "underline"=0, "strike through"=0, "font color"=16777216}, "error in (no error)"=w735) -> ("report out"=w738:refnum<class "NI_report.lvclass">, "error out"=w739:errorcluster)  [unwired: 8 in, 1 out]
            n299 = call-poly <vilib>:"Word Easy Table.vi"("report in"=w738, "column headers"=string[] ["框号", "长/mm", "宽/mm", "面积/mm2", "Z值/mm", "部位", "类型", "合格性"], "data"=w734, "error in (no error)"=w739) -> ("report out"=w733:refnum<class "NI_report.lvclass">, "error out"=w732:errorcluster)  [unwired: 9 in, 1 out]
          }
          frame #5 {
            n300 = local read "穿透图原始路径"() -> (w747:path)
            n301 = local read "报告模式"() -> (w745:string)
            n302 = Path To String(path=w747) -> (string=w751:string)
            n303 = String Length(string=w751) -> (length=w752:i32)
            n304 = Subtract(x=w752, y=4) -> (x-y=w753:i32)
            n305 = Concatenate Strings("_" ("字符串"), w745, "_.docx" ("字符串")) -> (w743:string)
            n306 = Replace Substring(3:w753, 4:w743, 5:w751) -> (1:w750:string)  [unwired: 1 in, 1 out]
            n307 = String To Path(string=w750) -> (path=w748:path)
            "添加的路径" <- w748
            n308 = call-dynamic "Save Report to File.vi"("report in"=w755, "report file path"=w748, "prompt to replace? (F)"=TRUE, "error in (no error)"=w754) -> ("report out"=w759:refnum<class "NI_report.lvclass">, "error out"=w758:errorcluster)  [unwired: 10 in]
            n309 = call <vilib>:"Word Bring to Front.vi"("report in"=w759, "window state (maximized)"=enum16{"maximized", "minimized", "normal"}."normal", "error in (no error)"=w758) -> ()  [unwired: 11 in, 2 out]
          }
          frame #6 {
            w760 = string[][] [] ("弥散类检测结果合并")
            n310 = local write "弥散类检测结果合并"(w760) -> ()
            n311 = local write "分层类检测结果合并"(w760) -> ()
            n312 = One Button Dialog(message="完成评定并退出程序！\n请查看word报告" ("消息")) -> ()  [unwired: 1 in, 1 out]
          }
        }
      }
      event "stop": Value Change {
        (unwired) 0
        # "退出软件"
        n313 = event-data() -> ("NewVal"=w764:bool)  [unwired: 1 in, 4 out]
        n314 = Two Button Dialog(message="是否关闭本软件？" ("消息")) -> (T button?=w765:bool)  [unwired: 2 in]
        n315 = And(x=w764, y=w765) -> (x .and. y?=w763:bool)
        n316 = case shown="真" w763 {
          frame False {
          }
          frame True {
            w766 = TRUE ("All Images? (No)")
            n317 = local read "穿透图"() -> (w768:T1)
            n318 = local read "反射图"() -> (w767:T1)
            n319 = call "IMAQ Dispose"("All Images? (No)"=w766, "Image"=w768) -> ()  [unwired: 4 in, 1 out]
            n320 = call "IMAQ Dispose"("All Images? (No)"=w766, "Image"=w767) -> ()  [unwired: 4 in, 1 out]
            n321 = disable-structure shown="RUN_TIME_ENGINE==True" {
              frame condition #0 {
                n322 = Quit LabVIEW() -> ()  [unwired: 1 in]
              }
              frame condition #1 (active) {
                n323 = Stop() -> ()  [unwired: 1 in]
              }
            }
          }
        }
      }
    }
    n324 = local read "模式选择"() -> (w46:u16)
    n325 = One Button Dialog(message="开始标注！\n全部标注完成后，\n请点击“完成标注”按钮" ("消息")) -> ()  [unwired: 1 in, 1 out]
    n326 = case shown="1" w46 {
      tunnel: w45 -> [w50 w120]
      tunnel: [w49 w119] -> w44
      frame 0, Default {
        w54 = i32[] [2] items=["No Event"=0, "Click Event"=1, "Draw Event"=2, "Size Event"=4, "Scroll Event"=5, "Double Click Event"=8] ("Which Events")
        # "循环的方式给输入图像手动画框"
        # "只对穿透图时画框的分支"
        n327 = local read "穿透图"() -> (w56:T1)
        n328 = invoke on="穿透图" class="ImageControl" method="Get Last Event"("Which Events"=w54) -> ("Type"=w52:i32)  [unwired: 7 in, 7 out]
        n329 = property on="穿透图" class="ImageControl"() -> ("ROI"=w53:T5)  [unwired: 2 in, 2 out]
        n330 = Not Equal To 0?(x=w52) -> (x != 0?=w51:bool)
        n331 = case shown="真" w51 {
          tunnel: w56 -> [w60 w72]
          tunnel: [w60 w71] -> w55
          tunnel: [w58 w69] -> w49
          tunnel: w50 -> [w58 w70]
          tunnel: w53 -> [_ w68]
          frame False {
            n332 = Wait (ms)(milliseconds to wait=u32 100 ("毫秒倍数")) -> ()  [unwired: 1 out]
            n333 = Wait (ms)(milliseconds to wait=u32 50) -> ()  [unwired: 1 out]
          }
          frame True {
            n334 = flat-sequence {
              tunnel: w72 -> [w73]
              tunnel: [w73] -> w67
              tunnel: w68 -> [w76]
              tunnel: [w76] -> w66
              tunnel: w70 -> [w75]
              tunnel: [w74] -> w65
              tunnel: w67 -> [w85]
              tunnel: w66 -> [w84]
              tunnel: w65 -> [w77]
              tunnel: [w87] -> w64
              tunnel: [w77] -> w63
              tunnel: [w81] -> w62
              tunnel: [w79] -> w61
              tunnel: w64 -> [w109]
              tunnel: w63 -> [w108]
              tunnel: w62 -> [w100]
              tunnel: w61 -> [w97]
              tunnel: [w109] -> w71
              tunnel: [w108] -> w69
              frame #0 {
                # "将当前ROI数据存入框组内"
                n335 = Build Array (concatenate)(w75, w76) -> (w74:T3)
              }
              frame #1 {
                # "在穿透图上画框"
                # "图层名Group与“框&图层计数”变量同名，\neg：1号框对应group1"
                # "overlay text在ROI的左上角添加计数显示"
                # "overlay ROI代表用户手画绿色框的图层添加"
                n336 = Unbundle(w84) -> ("Global Rectangle"=w92:i32[])  [unwired: 1 out]
                n337 = Array Size(array=w77) -> (size(s)=w79:i32)
                n338 = Number To Decimal String(number=w79) -> (decimal integer string=w80:string)  [unwired: 1 in]
                n339 = local write "框数"(w79) -> ()
                n340 = Index Array(array=w92, index=1 ("索引")) -> (element=w90:i32)
                n341 = Index Array(array=w92, index=0 ("索引")) -> (element=w91:i32)
                n342 = Concatenate Strings(w80, "#" ("字符串")) -> (w81:string)
                n343 = call "IMAQ Overlay ROI"("Group"=w81, "ROI Descriptor"=w84, "Image"=w85) -> ("Image Out"=w93:T1)  [unwired: 7 in, 1 out]
                n344 = Bundle(w91, w90) -> (w86:cluster{i32, i32})  [unwired: 1 in]
                n345 = local read "自定义字体"() -> (w83:T2)
                n346 = call "IMAQ Overlay Text"("Group"=w81, "Text Color (black)"=u32 16711680, "Font, Size & Style"=w83, "String"=w81, "Origin"=w86, "Image"=w93) -> ("Image Out"=w87:T1)  [unwired: 4 in, 1 out]
              }
              frame #2 {
                # "存放部位信息的1D数组，后续生成报告使用"
                # "0：位于蒙皮部位\n1：位于筋条部位"
                n347 = call "缺陷部位标注2"() -> ("位于筋条处"=w105:bool, "位于蒙皮处"=w104:bool)  [unwired: 16 in, 2 out]
                n348 = Build Array(w104, w105) -> (w106:bool[])
                n349 = Boolean Array To Number(Boolean array=w106) -> (number=w107:u32)
                n350 = case shown="1, 默认" w107 {
                  tunnel: ["蒙皮处" ("t") "筋条处" ("t")] -> w95
                  frame 1, Default {
                  }
                  frame 2 {
                  }
                }
                n351 = local read "部位信息"() -> (w99:string[])
                n352 = Decrement(x=w97) -> (x-1=w96:i32)
                n353 = Insert Into Array(array=w99, index=w96, new element=w95) -> (w98:string[])
                n354 = Concatenate Strings("框号为" ("字符串"), w100, "\n", "类别为" ("字符串"), w95) -> (w94:string)
                n355 = local write "连接的字符串"(w94) -> ()
                n356 = local write "部位信息"(w98) -> ()
              }
            }
          }
        }
        n357 = local write "穿透图"(w55) -> ()
        n358 = local write "框组"(w49) -> ()
      }
      frame 1 {
        w114 = i32[] [2] items=["No Event"=0, "Click Event"=1, "Draw Event"=2, "Size Event"=4, "Scroll Event"=5, "Double Click Event"=8] ("Which Events")
        # "对穿透图和反射图同时画框的分支"
        # "循环的方式给输入图像手动画框"
        n359 = local read "反射图"() -> (w117:T1)
        n360 = local read "穿透图"() -> (w112:T1)
        n361 = invoke on="穿透图" class="ImageControl" method="Get Last Event"("Which Events"=w114) -> ("Type"=w113:i32)  [unwired: 7 in, 7 out]
        n362 = Not Equal To 0?(x=w113) -> (x != 0?=w118:bool)
        n363 = case shown="假" w118 {
          tunnel: w112 -> [w124 w140]
          tunnel: [w124 w139] -> w116
          tunnel: [w121 w134] -> w119
          tunnel: w120 -> [w121 w138]
          tunnel: w117 -> [w123 w137]
          tunnel: [w123 w136] -> w115
          frame False {
            n364 = Wait (ms)(milliseconds to wait=u32 50 ("毫秒倍数")) -> ()  [unwired: 1 out]
          }
          frame True {
            n365 = property on="穿透图" class="ImageControl"() -> ("ROI"=w135:T5)  [unwired: 2 in, 2 out]
            n366 = flat-sequence {
              tunnel: w140 -> [w144]
              tunnel: [w144] -> w133
              tunnel: w135 -> [w145]
              tunnel: [w145] -> w132
              tunnel: w138 -> [w141]
              tunnel: w137 -> [w143]
              tunnel: [w143] -> w131
              tunnel: [w142] -> w130
              tunnel: w133 -> [w154]
              tunnel: w132 -> [w153]
              tunnel: w131 -> [w159]
              tunnel: w130 -> [w146]
              tunnel: [w160] -> w129
              tunnel: [w158] -> w128
              tunnel: [w146] -> w127
              tunnel: [w150] -> w126
              tunnel: [w148] -> w125
              tunnel: w129 -> [w183]
              tunnel: w128 -> [w182]
              tunnel: w127 -> [w181]
              tunnel: w126 -> [w172]
              tunnel: w125 -> [w169]
              tunnel: [w183] -> w139
              tunnel: [w182] -> w136
              tunnel: [w181] -> w134
              frame #0 {
                # "将当前ROI数据存入框组内"
                n367 = Build Array (concatenate)(w141, w145) -> (w142:T3)
              }
              frame #1 {
                w156 = u32[] [15663114] ("Colors (Green)")
                w152 = u32 16711776 ("Text Color (black)")
                # "在反射图上对应位置画框"
                # "在穿透图上画框"
                # "图层名Group与“框&图层计数”变量同名，\neg：1号框对应group1"
                # "overlay text在ROI的左上角添加计数显示"
                # "overlay ROI代表用户手画绿色框的图层添加"
                n368 = Array Size(array=w146) -> (size(s)=w148:i32)
                n369 = Unbundle(w153) -> ("Global Rectangle"=w165:i32[])  [unwired: 1 out]
                n370 = Number To Decimal String(number=w148) -> (decimal integer string=w149:string)  [unwired: 1 in]
                n371 = local write "框数"(w148) -> ()
                n372 = Concatenate Strings(w149, "#" ("字符串")) -> (w150:string)
                n373 = Index Array(array=w165, index=1 ("索引")) -> (element=w163:i32)
                n374 = Index Array(array=w165, index=0 ("索引")) -> (element=w164:i32)
                n375 = local read "自定义字体"() -> (w151:T2)
                n376 = call "IMAQ Overlay ROI"("Colors (Green)"=w156, "Group"=w150, "ROI Descriptor"=w153, "Image"=w154) -> ("Image Out"=w166:T1)  [unwired: 6 in, 1 out]
                n377 = call "IMAQ Overlay ROI"("Colors (Green)"=w156, "Group"=w150, "ROI Descriptor"=w153, "Image"=w159) -> ("Image Out"=w157:T1)  [unwired: 6 in, 1 out]
                n378 = Bundle(w164, w163) -> (w155:cluster{i32, i32})  [unwired: 1 in]
                n379 = call "IMAQ Overlay Text"("Group"=w150, "Text Color (black)"=w152, "Font, Size & Style"=w151, "String"=w150, "Origin"=w155, "Image"=w157) -> ("Image Out"=w158:T1)  [unwired: 4 in, 1 out]
                n380 = call "IMAQ Overlay Text"("Group"=w150, "Text Color (black)"=w152, "Font, Size & Style"=w151, "String"=w150, "Origin"=w155, "Image"=w166) -> ("Image Out"=w160:T1)  [unwired: 4 in, 1 out]
              }
              frame #2 {
                # "存放部位信息的1D数组，后续生成报告使用"
                # "0：位于蒙皮部位\n1：位于筋条部位"
                n381 = call "缺陷部位标注"() -> ("位于筋条处"=w177:bool, "位于蒙皮处"=w176:bool)  [unwired: 16 in, 2 out]
                n382 = Build Array(w176, w177) -> (w178:bool[])
                n383 = Boolean Array To Number(Boolean array=w178) -> (number=w179:u32)
                n384 = local read "部位信息"() -> (w171:string[])
                n385 = case shown="1, 默认" w179 {
                  tunnel: ["蒙皮处" ("t") "筋条处" ("t")] -> w167
                  frame 1, Default {
                  }
                  frame 2 {
                  }
                }
                n386 = Decrement(x=w169) -> (x-1=w168:i32)
                n387 = Insert Into Array(array=w171, index=w168, new element=w167) -> (w170:string[])
                n388 = Concatenate Strings("框号为" ("字符串"), w172, "\n", "类别为" ("字符串"), w167) -> (→"连接的字符串":string)
                n389 = local write "部位信息"(w170) -> ()
              }
            }
          }
        }
        n390 = local write "框组"(w119) -> ()
        n391 = local write "穿透图"(w116) -> ()
        n392 = local write "反射图"(w115) -> ()
      }
    }
    n393 = local read "stop"() -> (w43:bool)
    n394 = Or(x=w42, y=w43) -> (x .or. y?=w41:bool)
  }
  n395 = disable-structure shown="禁用" {
    frame Disabled {
      n396 = while {
        stop <- FALSE stop-if-true
        n397 = local read "删除标注"() -> (w772:bool)
        n398 = local read "查看标注"() -> (w771:bool)
        n399 = Or(x=w772, y=w771) -> (x .or. y?=w773:bool)
        n400 = local write "开始标注"(w773) -> ()
        n401 = Wait Until Next ms Multiple(millisecond multiple=u32 50 ("毫秒倍数")) -> ()  [unwired: 1 out]
      }
    }
    frame Enabled {
    }
  }
  "临界面积百分比值" <- w3
  "输入的灰度阈值" <- w4
